vi "Main.vi"() -> ()   [LabVIEW 2023, in "QSM - Main.lvlib"]
uses:
  QSM - Main.lvlib
  Sched and Tubes.vi
  QSM - IODocs/IO Docs.vi
  LIMITS.vi
  QSM - Alarms/ALARMS.vi
  Controls/State Machine Message.ctl
  Controls/Message Queue Element Position.ctl
  UserCredentials.ctl
  Controls/biasdiff.ctl
  Controls/Event Handler Message.ctl
  <vilib>/event_ctls.llb/usereventprio.ctl
  QSM - Alarms/QSM - Alarms.lvlib
  QSM - IODocs/QSM - IODocs.lvlib
  Controls/gridvals.ctl
  QSM - Editor/QSM - Editor.lvlib
  QSM - Limits/QSM - Limits.lvlib
  Status.ctl
  Schedule.ctl
  Controls/stepvariables.ctl
  Controls/remoterdgs.ctl
  Controls/pulserdgs.ctl
  Controls/pulseparams.ctl
  Controls/cammeasures.ctl
  Controls/camdeflections.ctl
  Controls/camrefvals.ctl
  Controls/camexpvals.ctl
  Controls/camsettings.ctl
panel:
  out "Status 2":string="No Error"
  in  "PrintDatasheet":bool
  out "Status":T1
  out "Retest Select":bool[](array[boolean])
  out "Retest Step":u8
  in  "RetestEnd":bool
  in  "RetestOne":bool
  in  "FPCamera_PB":bool
  out "AIO Array Temp":dbl[](array[numeric])
  out "camsettings":T2
  out "current time":timestamp
  out "camrefs":T3
  out "deflections":T4
  out "cam measures":T5
  out "camexpvals":T6
  out "pulse params":T7
  out "pulse readings":T8
  out "Running":bool
  out "Sched Loaded":bool
  out "Tube Loaded":bool
  in  "Digital IO":bool[](array[boolean])
  out "Analog IO":dbl[](array[numeric])
  out "OffsetGain":dbl[](array[numeric])
  out "remrdgs":T9
  in  "Param Gx Only":cluster{"P06 G1 ONLY":bool, "P21 G2 ONLY":bool}
  in  "GXVALS":T10 {"g2rdggain" step=1e-05; "g2rdgoffset" step=1e-05; "g2spgain" step=1e-05; "g2spoffset" step=1e-05; "g1rdggain" step=1e-05; "g1rdgoffset" step=1e-05; "g1spgain" step=1e-05; "g1spoffset" step=1e-05}
  in  "BIAS DIFF":T11 {"DIFF" step=10.0; "BIAS" step=10.0}
  out "LIMITS":sgl[](array[numeric])
  in  "Run Results":i32(listbox)
  out "ALARM":bool
  out "PROC NOK":bool
  out "ALARMS":bool[](array[boolean])
  out "PROC OK":bool[](array[boolean])=[TRUE]
  out "STEP VARS":T12
  in  "PLC CURRENT STEP":u16 max=32
  in  "RESET Button":bool
  in  "RUN Button":bool
  in  "FINAL STEP":u16 max=32
  out "CURRENT STEP":u16 max=32
  in  "FIRST STEP":u16 max=32
  in  "ALARMS BUtton":bool
  in  "LIMITS Button":bool
  in  "IO/DOCS Button":bool
  in  "ENTER OP":string
  in  "ENTER SN":string
  in  "View Sched Button":bool
  in  "Schedule":T13 caption="Multicolumn Listbox"
  out "SchedNames[]":string[](array[string])
  out "SchedName":string
  out "SchedNum":string
  in  "sched sel Button":bool
  out "schd61-80":u32
  out "schd31-60":u32
  out "schd1-30":u32
  out "AP%":dbl
  out "T10":dbl
  out "T100":dbl
  out "HS":dbl
  out "RTC":dbl
  out "NAME":string
  out "TUBE":dbl
  in  "Load Tube Button":bool
  in  "Error In":errorcluster
  out "Error Out":errorcluster
  in  "Security Button":bool
  in  "stop":bool
  out "Access":u16
  out "Op Name":string
  out "BADGE NUMBER":string
  in  "Log In Button":bool
  in  "Editor Button":bool
  in  "User Creds":T14
  # "--STEP VARIABLES--"
  # "--CONTROLS--"
  # "--GRID TANK VALUES--"
  # "MCS-2093 Grid Tank\nFocal Spot Test Setup"
  # "XT229"
  # "ENTER SN"
  # "--CAMERA INTERFACE--"
  # "ENTER OP"
  # "REF"
  # "--READINGS--"
  # "Width"
  # "FrameRate"
  # "Mode"
  # "Length"
  # "--PULSE READINGS--"
  # "FW%max"
  # "X"
  # "Z"
  # "Y"
  # "MAG"
  # "pk"
  # "--STATUS--"
  # "**This Button Relaunches \nFLATPANELCAMERA application \nin event of crash/closure."
  # "OBpk"
  # "**Double Click Results Row \nto Select Retest Step**"
  # "FOCAL SPOT GRID TANK RUN RESULTS"
  # "OFFSET"
  # "OFFSET"
  # "GAIN"
  # "GAIN"
  # "OFFSET"
  # "OFFSET"
  # "GAIN"
  # "GAIN"
  # "STEP"
  # "NAME"
  # "NOTES"
  # "PARAMS"
  # "KV SP"
  # "MA/IF SP"
  # "EXP sec SP"
  # "COOL sec SP"
  # "scans.Mode"
  # "data item"
  # "min"
  # "max"
  # "init BIAS SP"
  # "init DIFF SP"
  # "max Gx"
  # "init EfDr SP"
  # "max Tries"
  # "TEST"
  # "LIM1"
  # "LIM2"
  # "LIM4"
  # "LIM3"
  # "CHAIN SCHEDS"
  # "RPTS"
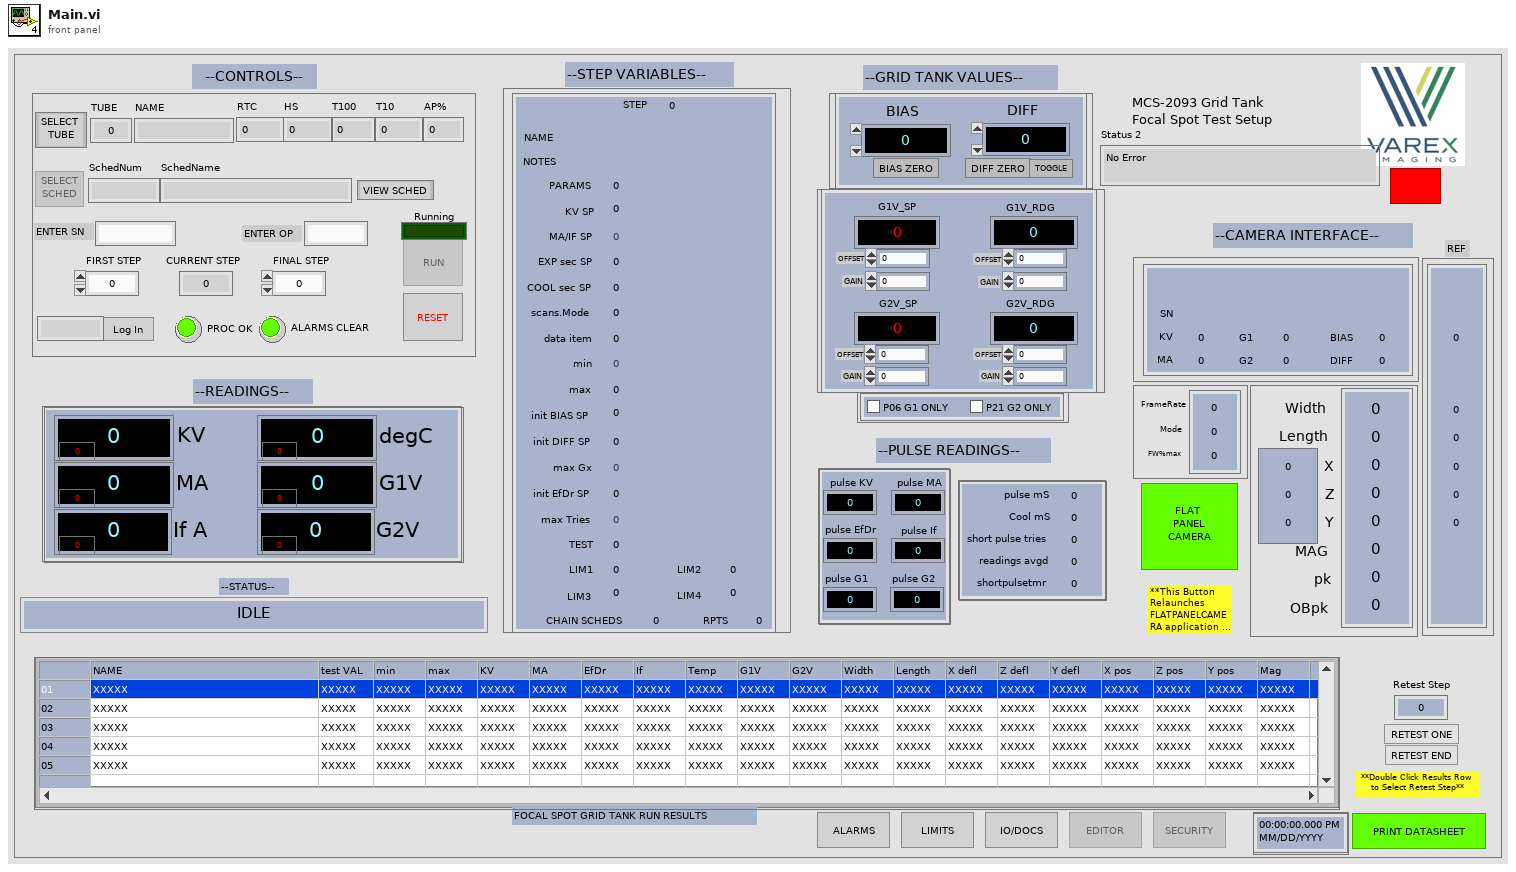
[diagram p1: front panel]
types:
  T1 = typedef "Status.ctl" = enum16{"IDLE", "RUN INITIATED", "RUNNING", "RESET INITIATED", "RESET", "RETESTING SELECTED STEP ONLY", "RETESTING SELECTED STEP TO END", "CAPTURING IMAGE", "WAITING FOR GRID SUPPLY", "WAITING FOR IMAGE", "ALARMS ACTIVE", "PROCNOK ACTIVE", "USER SIGNED ON", "TUBE SELECTED", "SCHEDULE SELECTED", "PRINTING DATASHEET", ""}
  T2 = typedef "QSM - Main.lvlib/camsettings.ctl" = cluster{"cam_FRAME_RATE":dbl, " cam_Mode":dbl, "cam_PERCENT_MAX":dbl}
  T3 = typedef "QSM - Main.lvlib/camrefvals.ctl" = cluster{"BIAS_ref":dbl, "cam_Wref":dbl, "cam_Lref":dbl, "cam_Xref":dbl, "cam_Zref":dbl, "cam_Yref":dbl}
  T4 = typedef "QSM - Main.lvlib/camdeflections.ctl" = cluster{"X_defl":dbl, "Y_defl":dbl, "Z_defl":dbl}
  T5 = typedef "QSM - Main.lvlib/cammeasures.ctl" = cluster{"cam_WIDTH":dbl, "cam_LENGTH":dbl, "cam_Xpos":dbl, "cam_Zpos":dbl, "cam_Ypos":dbl, "cam_MAG":dbl, "cam_PEAK":dbl, "cam_OB_pk":dbl}
  T6 = typedef "QSM - Main.lvlib/camexpvals.ctl" = cluster{"cam_IMAGE_PATH":string, "SN":string, "KV":dbl, "MA":dbl, "G1":dbl, "G2":dbl, "BIAS":dbl, "DIFF":dbl}
  T7 = typedef "QSM - Main.lvlib/pulseparams.ctl" = cluster{"pulse mS":dbl, "Cool mS":dbl, "short pulse tries":dbl, "readings avgd":dbl, "shortpulsetmr":dbl}
  T8 = typedef "QSM - Main.lvlib/pulserdgs.ctl" = cluster{"pulse EfDr":dbl, "pulse G1":dbl, "pulse G2":dbl, "pulse KV":dbl, "pulse MA":dbl, "pulse If":dbl}
  T9 = typedef "QSM - Main.lvlib/remoterdgs.ctl" = cluster{"remKVrdg":dbl, "remMArdg":dbl, "remIfArdg":dbl, "Temprdg":dbl, "G1Vrdg":dbl, "G2Vrdg":dbl, "remKVsp":dbl, "remMAsp":dbl, "remIfAsp":dbl, "Tempsp":dbl, "G1Vsp":dbl, "G2Vsp":dbl}
  T10 = typedef "QSM - Main.lvlib/gridvals.ctl" = cluster{"G1V_SP":dbl, "G2V_SP":dbl, "G1V_RDG":dbl, "G2V_RDG":dbl, "g1spoffset":dbl, "g1spgain":dbl, "g1rdgoffset":dbl, "g1rdggain":dbl, "g2spoffset":dbl, "g2spgain":dbl, "g2rdgoffset":dbl, "g2rdggain":dbl}
  T11 = typedef "QSM - Main.lvlib/biasdiff.ctl" = cluster{"BIAS":dbl, "BIAS_ZER":bool, "DIFF_ZER":bool, "DIFF_TOGGLE":bool, "DIFF":dbl}
  T12 = typedef "QSM - Main.lvlib/stepvariables.ctl" = cluster{"NAME":string, "NOTES":string, "PARAMS":u32, "KV  SP":dbl, "MA/IF  SP":dbl, "init BIAS SP":dbl, "max Gx":dbl, "TEST":u32, "min":dbl, "max":dbl, "LIM1":dbl, "LIM2":dbl, "LIM3":dbl, "LIM4":dbl, "data item":dbl, "chain scheds":dbl, "REPEATS":dbl, "STEP NUM":u32, "EXP s SP":dbl, "COOL s SP":dbl, "scans mode":dbl, "init EfDr":dbl, "max Tries":dbl, "init DIFF SP":dbl}
  T13 = typedef "Schedule.ctl" = i32
  T14 = typedef "UserCredentials.ctl" = cluster{"Badge Number":string, "Name":string, "Access":enum16{"", "Operator", "Admin", "Engineer"}}
  T15 = typedef "QSM - Main.lvlib/State Machine Message.ctl" = enum16{"Initialize", "Operator Signon", "Editor", "Security", "Select Tube", "Select Sched", "View Sched", "View IO/DOCS", "New Gx Val", "View LIMITS", "View ALARMS", "Start Step Change", "New Serial Number", "RUN Initiated", "RESET Initiated", "PLC Step Change", "RunResultRetestSelect", "Retest One", "Retest End", "PROC OK CHECK", "PROC NOK", "APIProcNOKUpdate", "APIAlarmsUpdate", "APILimitUpdate", "APIOperatorUpdate", "APIAnalogIOUpdate", "APIOffsetGainUpdate", "APIGXValsUpdate", "APIBiasDiffUpdate", "API Update Selected Tube", "API Update Selected Schedule", "ALARM CHECK", "ALARM ACTIVE", "CHECKS", "Print Datasheet", "FlatPanelCamera", "BIAS ZER", "DIFF ZER", "DIFF TOGGLE", "Handle Error", "Exit"}
  T16 = typedef "QSM - Main.lvlib/User Event Reference.ctl" = refnum<user-event>
  T17 = typedef "QSM - Main.lvlib/User Event Registration Reference.ctl" = refnum<event-registration>
  T18 = cluster{"Address IP":string, "Rack":i32, "Slot ":i32, "DB Number":i32, "Start":i32, "Amount":i32, "Word Length":i32}
  T19 = enum8{"Enabled", "Disabled", "Disabled and Grayed Out"}
  T20 = typedef "QSM - Main.lvlib/Message Queue Element Position.ctl" = enum16{"Front", "Back"}
  T21 = cluster{"Address IP":string, "Rack":i32, "Slot ":i32, "DB Number":i32, "Start":i32, "Amount":i32}
  T22 = typedef "usereventprio.ctl" = enum32{"high priority", "normal priority"}
  T23 = typedef "QSM - Main.lvlib/Event Handler Message.ctl" = enum16{"Exit"}
  T24 = cluster{"[0]":dbl, "[1]":dbl, "[2]":dbl, "[3]":dbl, "[4]":dbl, "[5]":dbl, "[6]":dbl, "[7]":dbl, "[8]":dbl, "[9]":dbl, "[10]":dbl, "[11]":dbl}
  T25 = cluster{"NAME":string, "NOTES":string, "PARAMS":u32, "KV  SP":dbl, "MA/IF  SP":dbl, "init BIAS SP":dbl, "max Gx":dbl, "TEST":u32, "min":dbl, "max":dbl, "LIM1":dbl, "LIM2":dbl, "LIM3":dbl, "LIM4":dbl, "data item":dbl, "chain scheds":dbl, "REPEATS":dbl, "STEP NUM":u32, "EXP s SP":dbl, "COOL s SP":dbl, "scans mode":dbl, "init EfDr":dbl, "max Tries":dbl, "init DIFF SP":dbl}
  T26 = cluster{"[0]":dbl, "[1]":dbl, "[2]":dbl, "[3]":dbl, "[4]":dbl, "[5]":dbl, "[6]":dbl, "[7]":dbl}
  T27 = enum32{"Bad", "Idle", "Run top level", "Running"}
  T28 = cluster{"Value[0]":dbl, "Value[1]":dbl, "Value[2]":dbl, "Value[3]":dbl, "Value[4]":dbl, "Value[5]":dbl, "Value[6]":dbl, "Value[7]":dbl, "Value[8]":dbl, "Value[9]":dbl, "Value[10]":dbl}
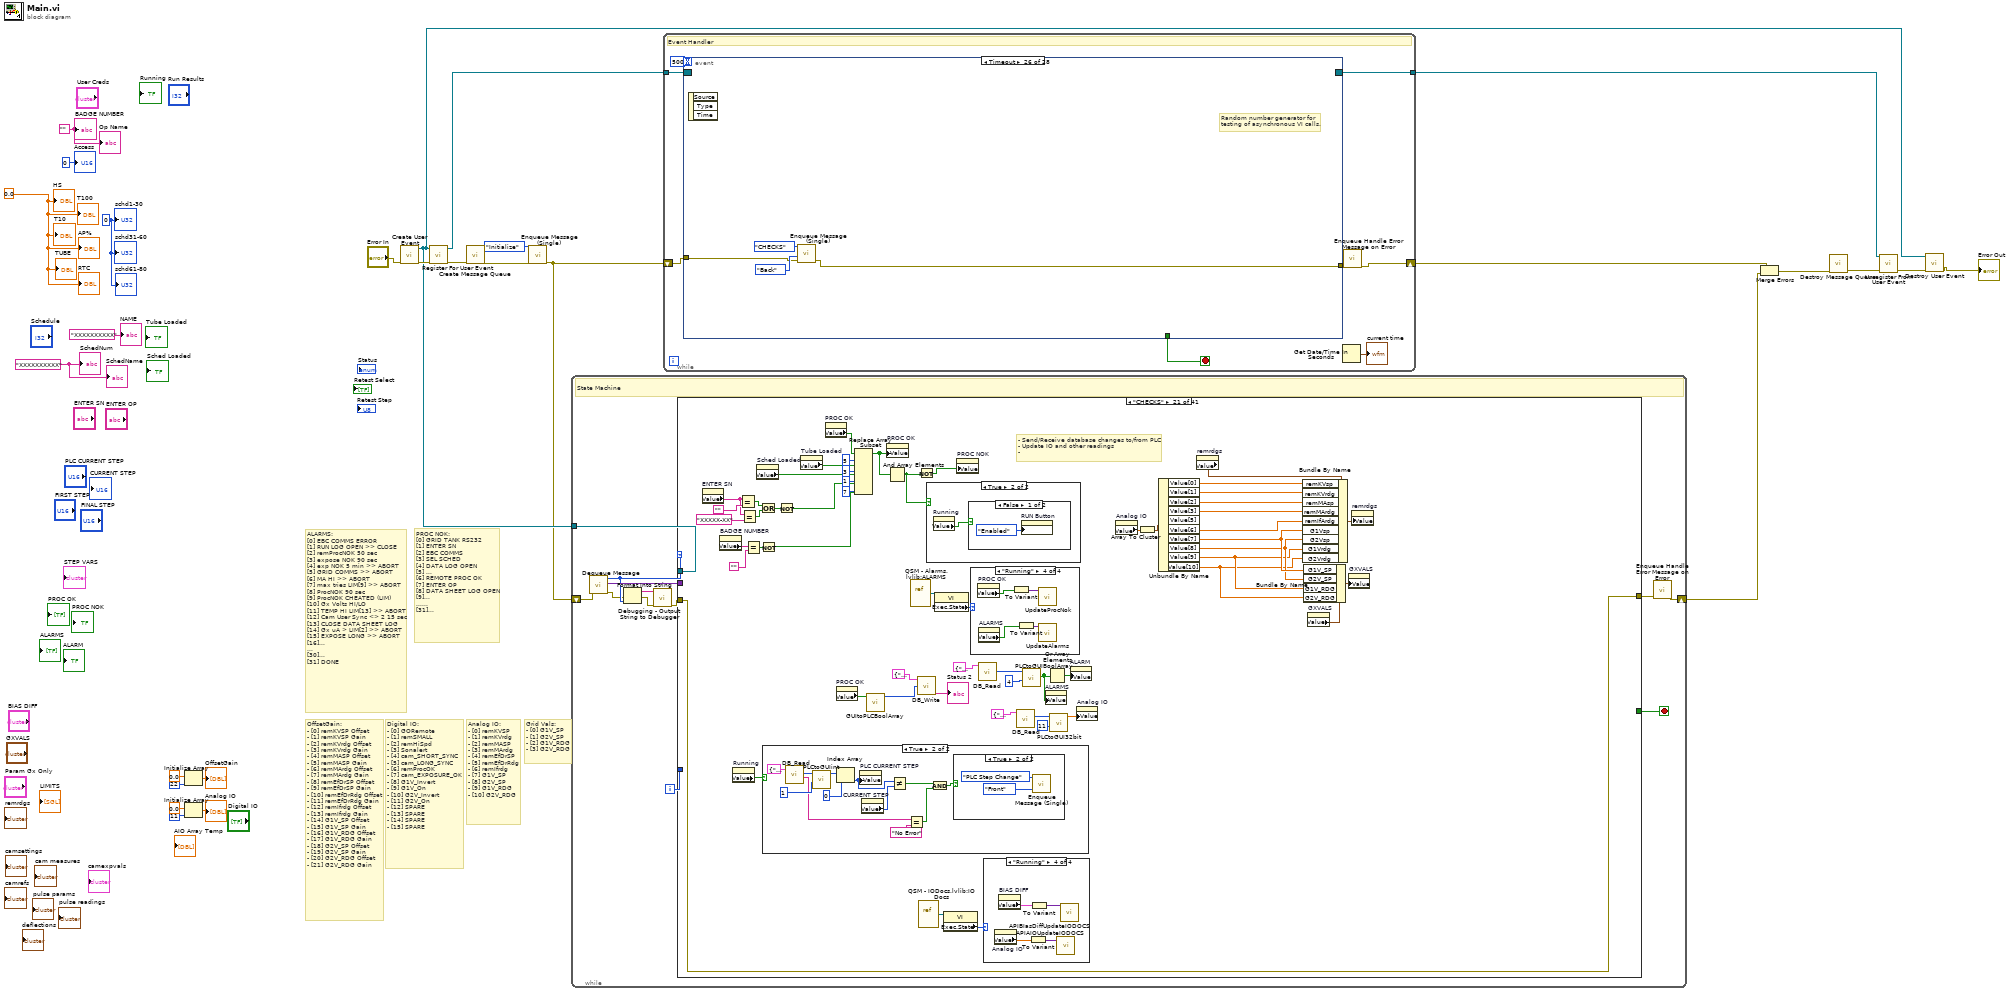
[diagram p0: block diagram]
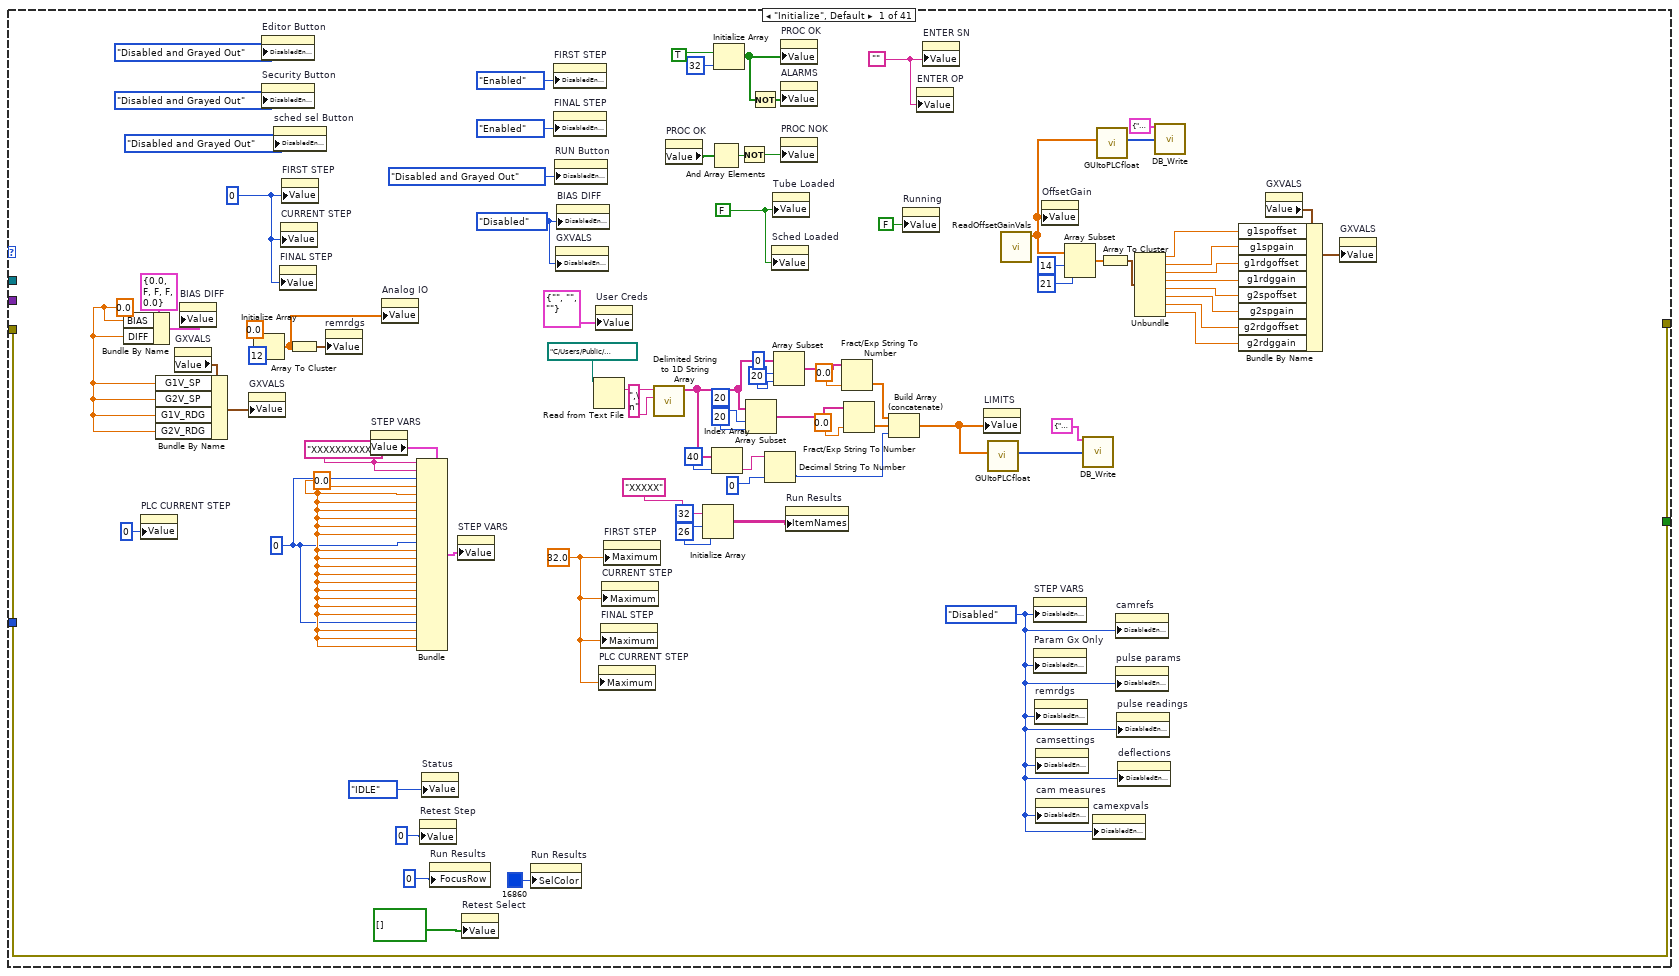
[diagram p2: hidden frame]
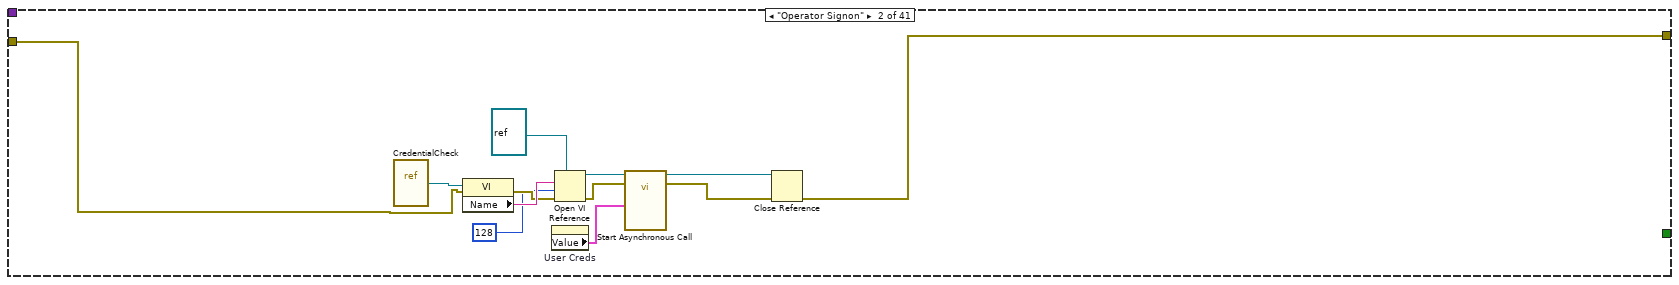
[diagram p3: hidden frame]
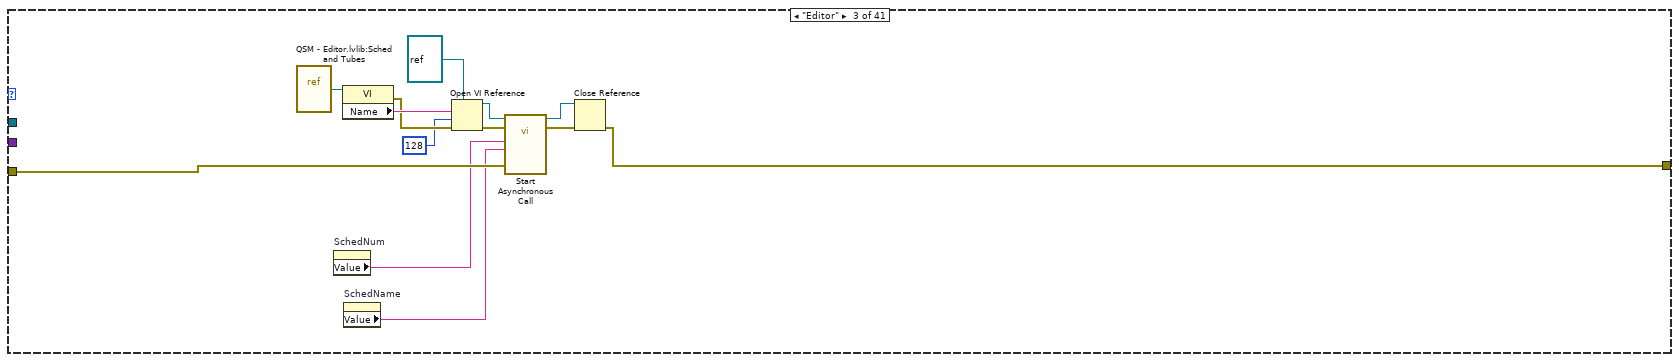
[diagram p4: hidden frame]
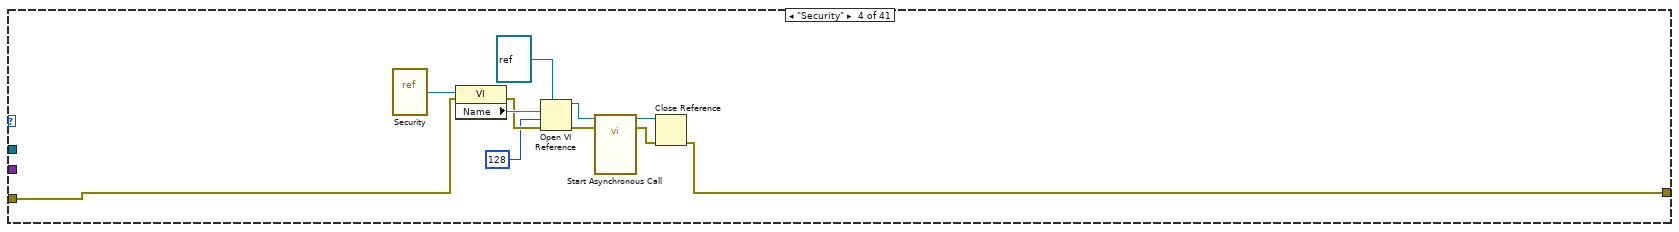
[diagram p5: hidden frame]
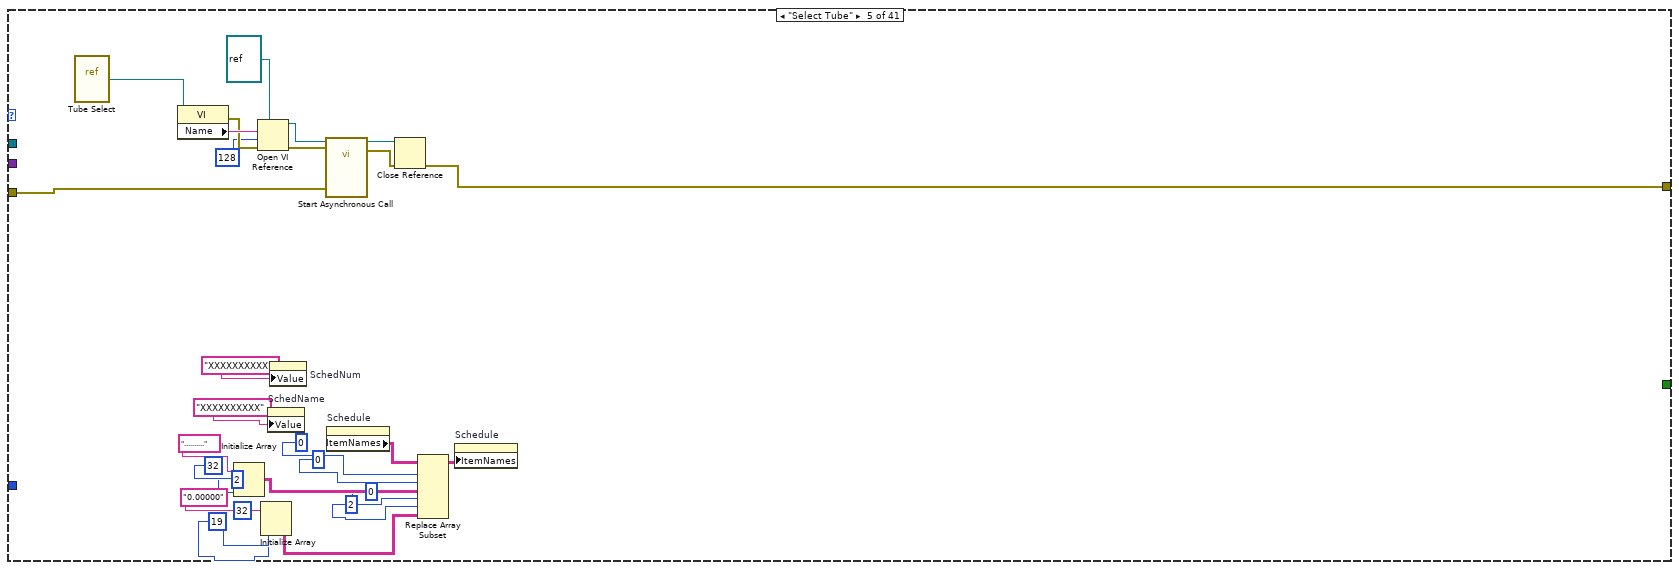
[diagram p6: hidden frame]
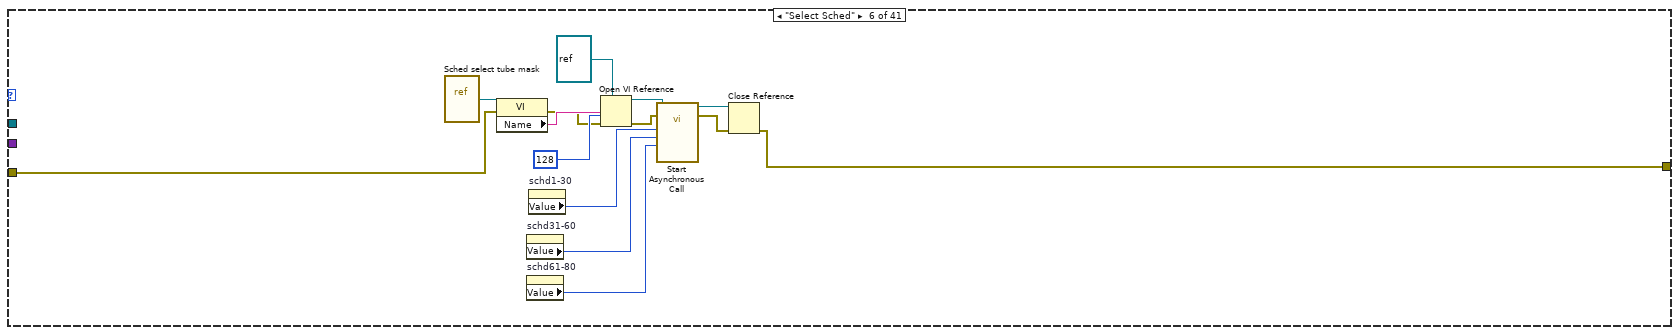
[diagram p7: hidden frame]
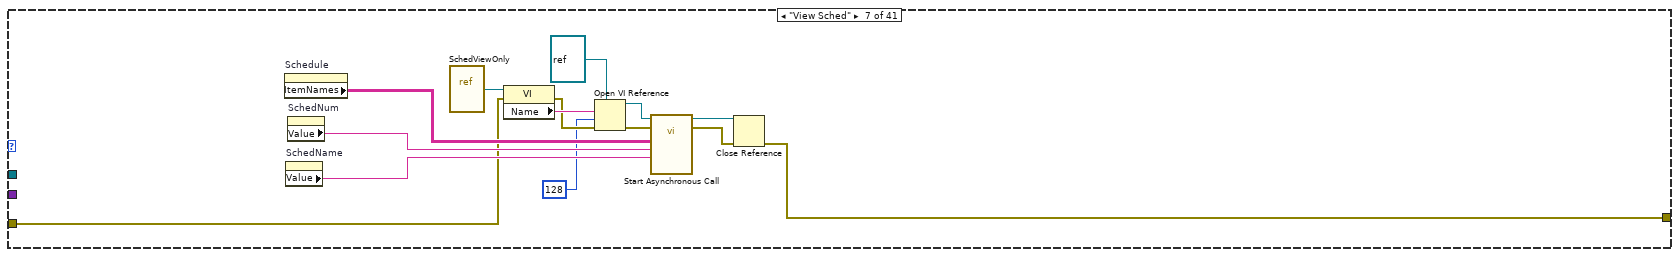
[diagram p8: hidden frame]
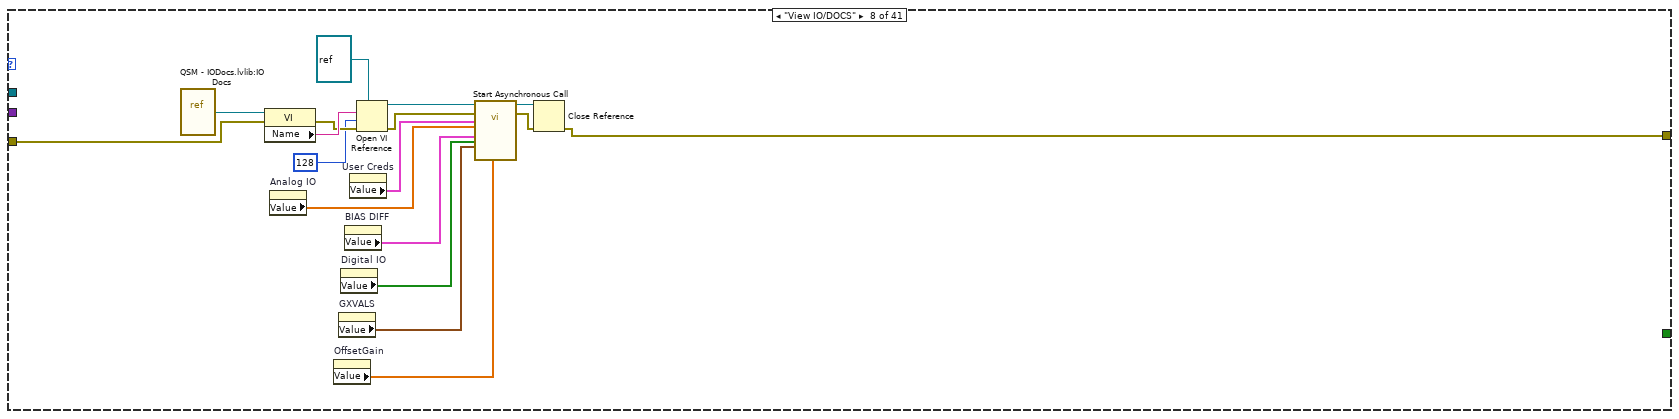
[diagram p9: hidden frame]
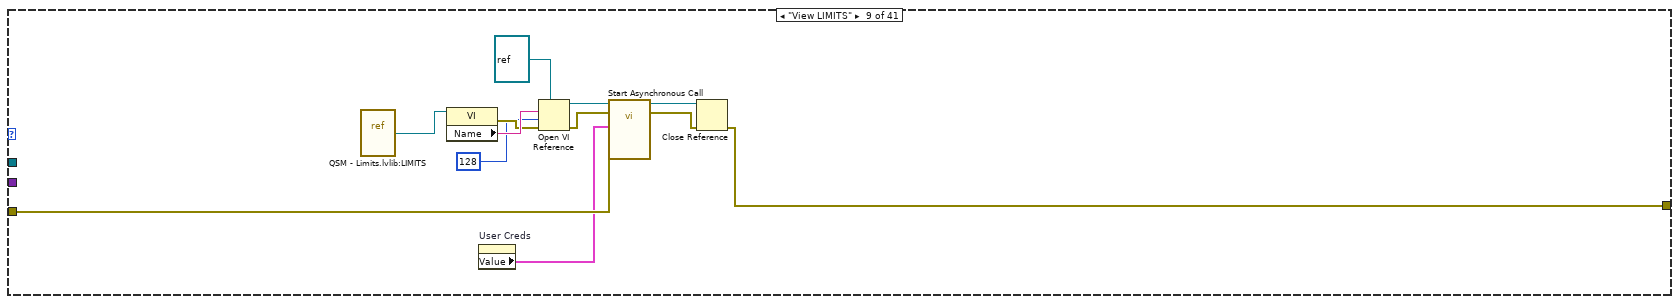
[diagram p10: hidden frame]
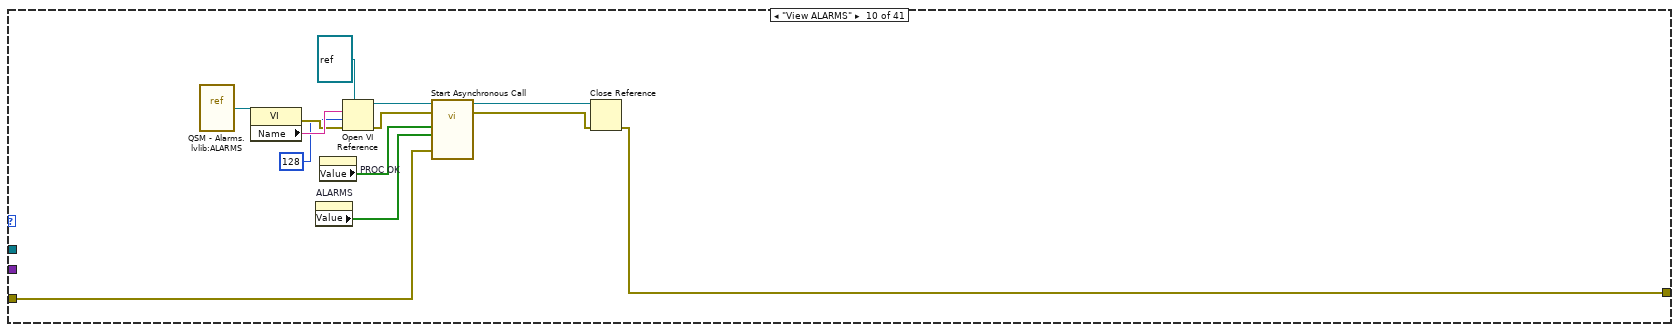
[diagram p11: hidden frame]
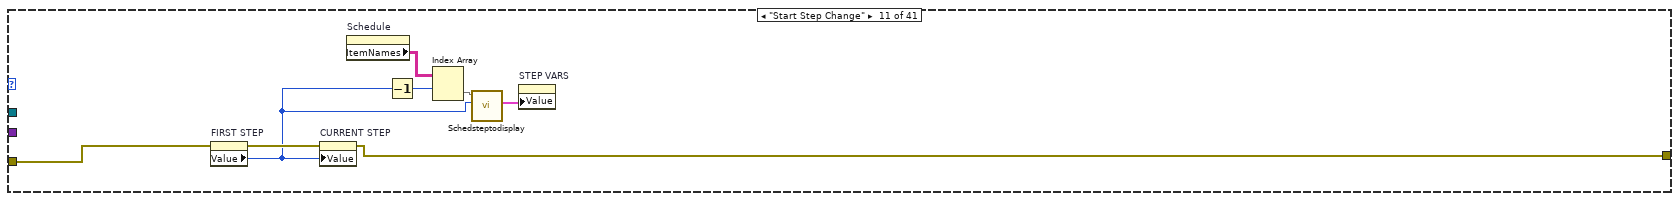
[diagram p12: hidden frame]
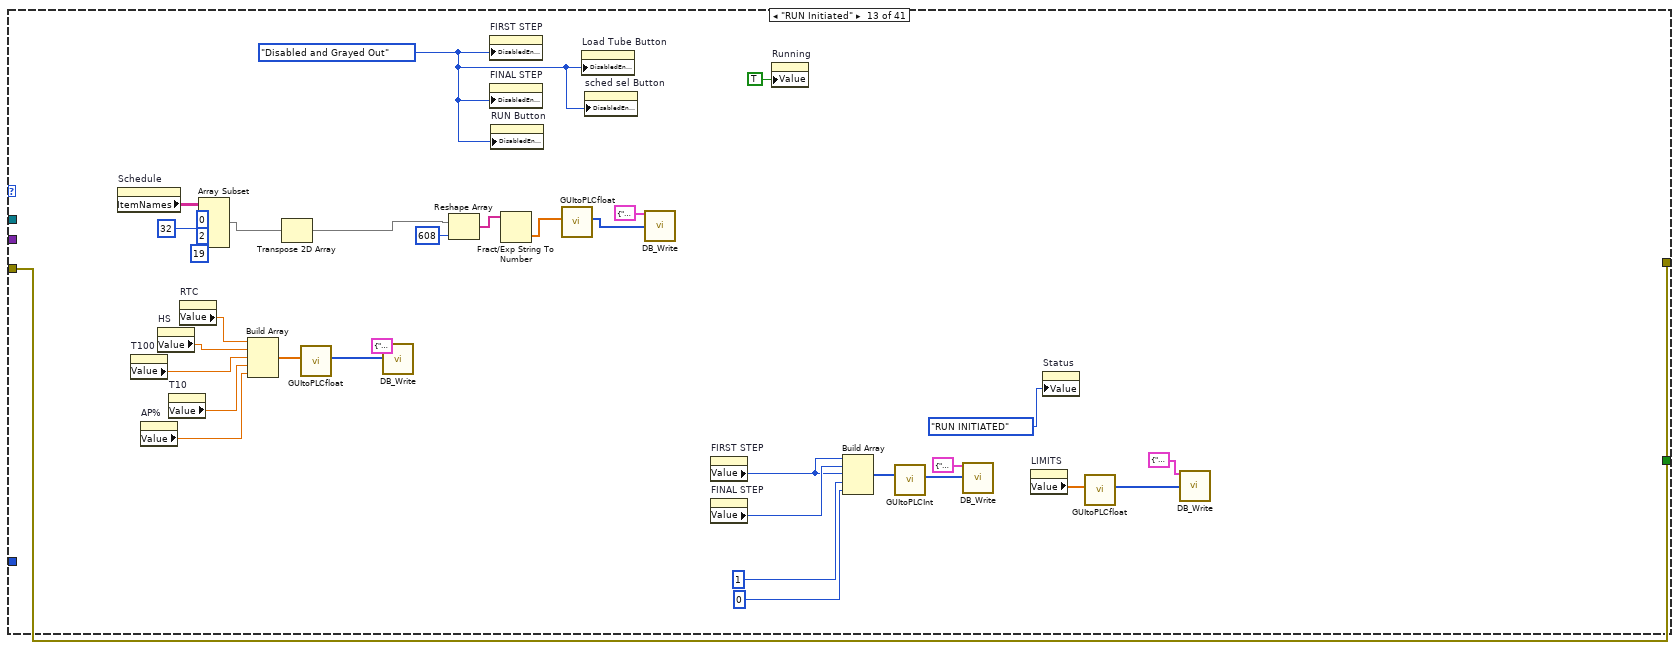
[diagram p14: hidden frame]
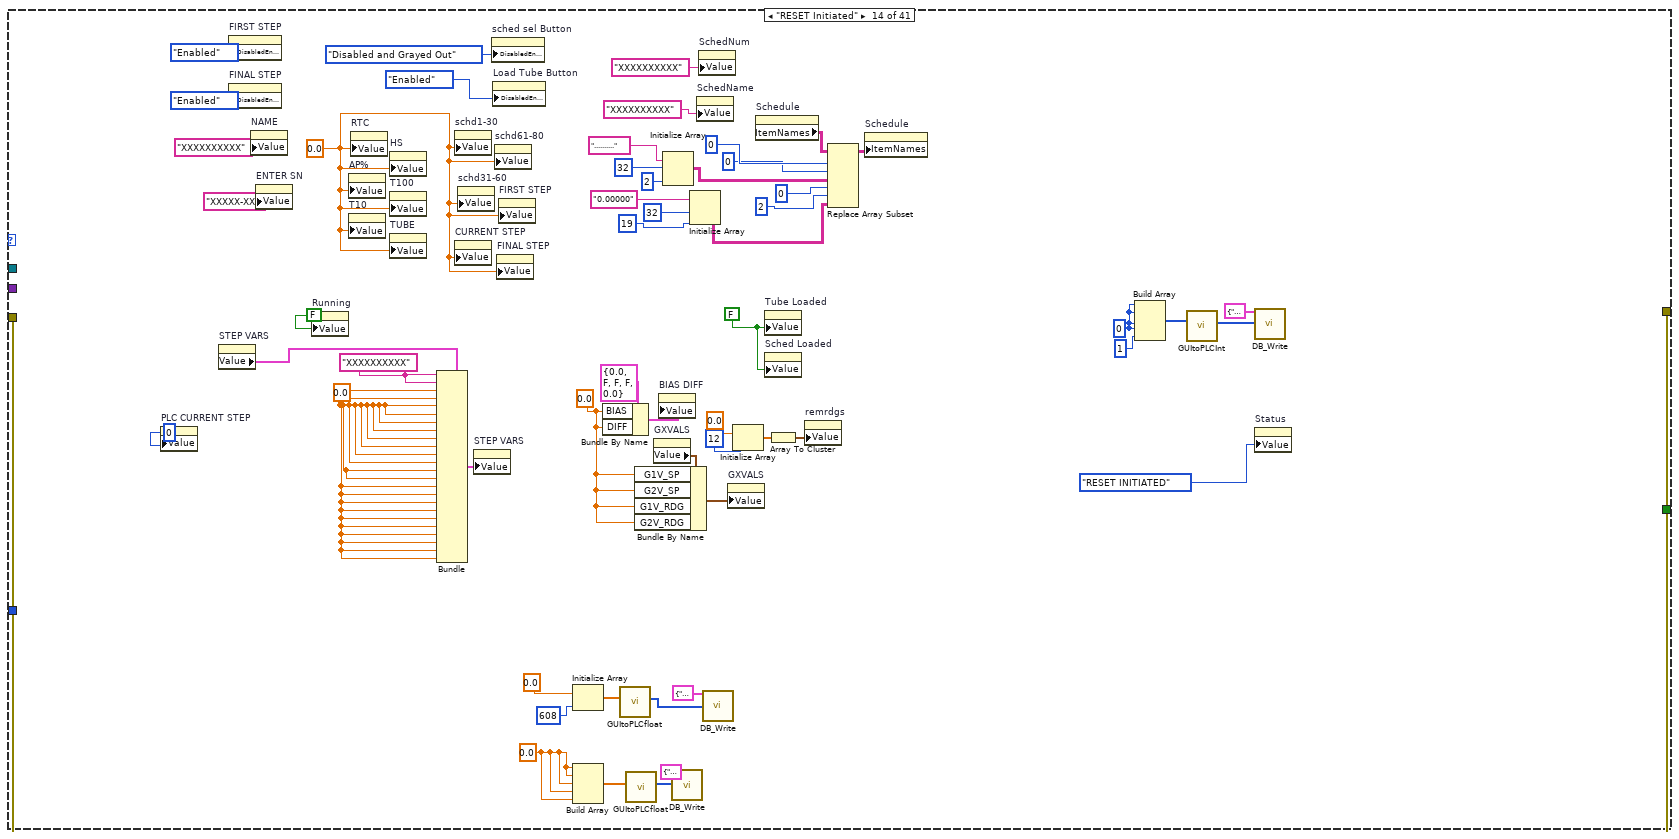
[diagram p15: hidden frame]
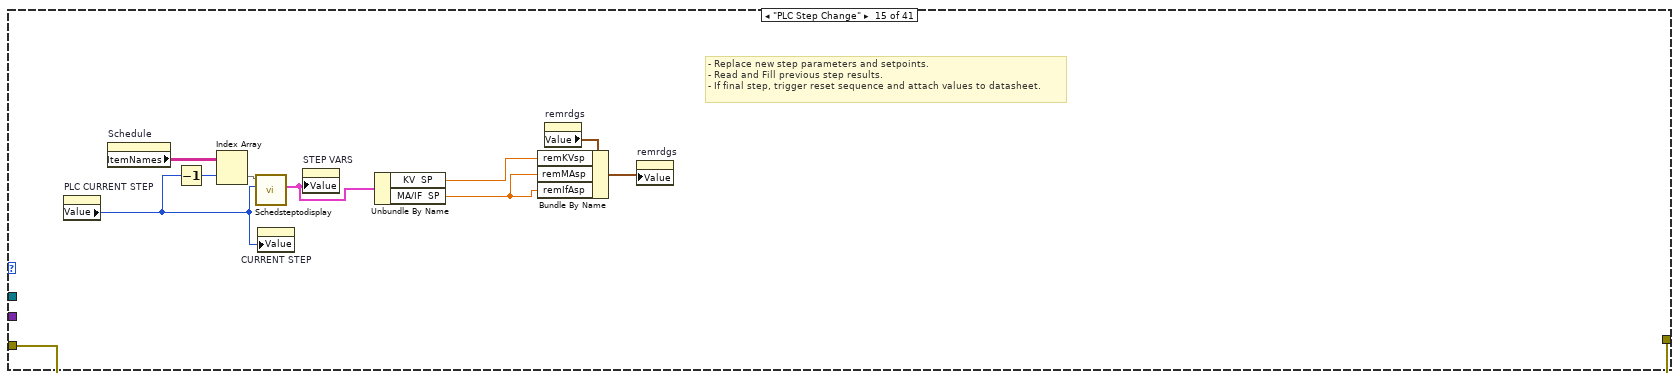
[diagram p16: hidden frame]
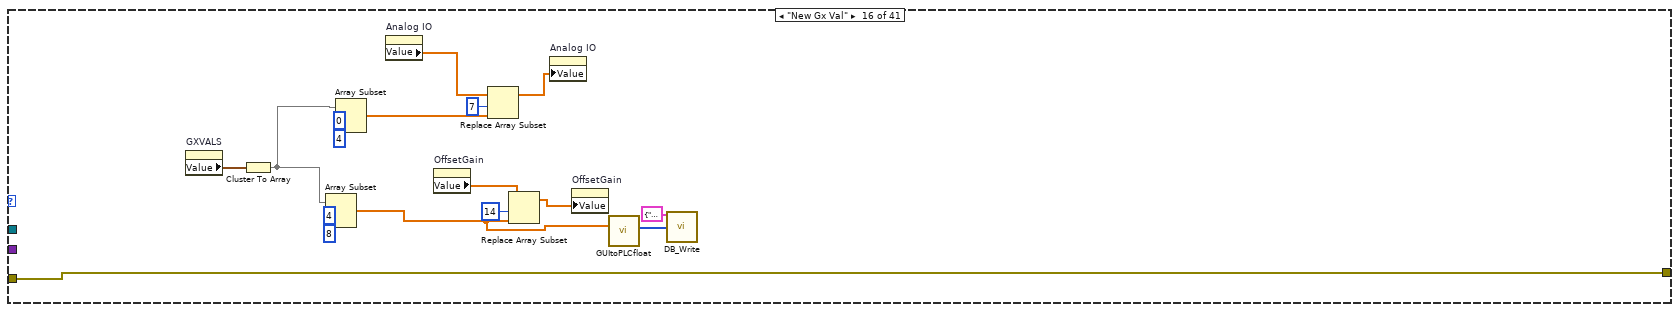
[diagram p17: hidden frame]
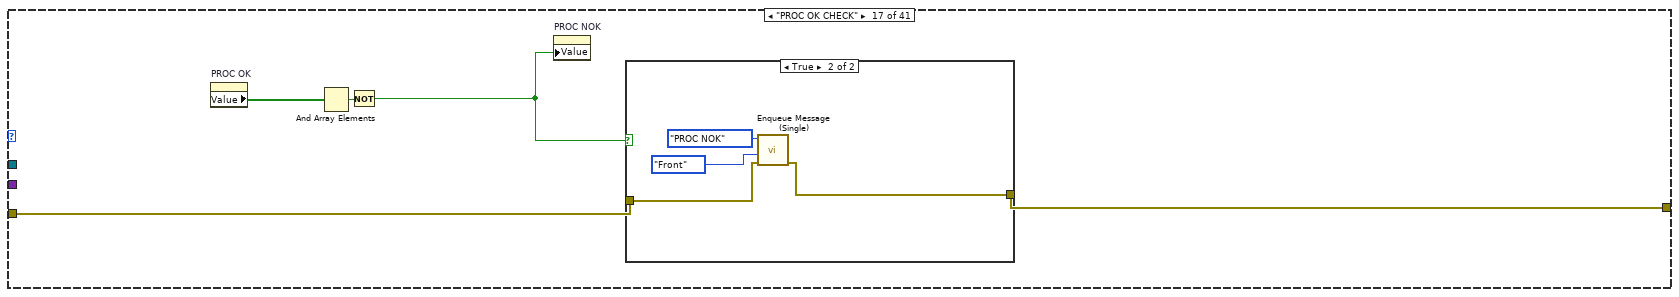
[diagram p18: hidden frame]
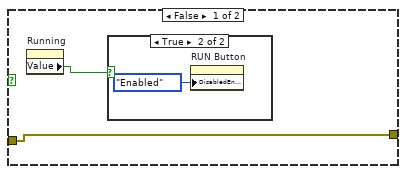
[diagram p19: hidden frame]
diagram:
  w18 = "XXXXXXXXXX" ("SchedNum")
  w19 = u32 0 ("schd1-30")
  w20 = 0.0 ("HS")
  w27 = "" ("Badge Number")
  # "Analog IO:\n- [0] remKVSP\n- [1] remKVrdg\n- [2] remMASP\n- [3] remMArdg\n- [4] remEfDrSP\n- [5] remEfDrRdg\n- [6] remIfrdg\n- [7] G1V_SP\n- [8] G2V_SP\n- [9] G1V_RDG\n- [10] G2V_RDG"
  # "OffsetGain:\n- [0] remKVSP Offset\n- [1] remKVSP Gain\n- [2] remKVrdg Offset\n- [3] remKVrdg Gain\n- [4] remMASP Offset\n- [5] remMASP Gain\n- [6] remMArdg Offset\n- [7] remMArdg Gain\n- [8] remEfDrSP Offset\n- [9] remEfDrSP Gain\n- [10] remEfDrRdg Offset\n- [11] remEfDrRdg Gain\n- [12] remIfrdg Offset\n- [13] remIfrdg Gain\n- [14] G1V_SP Offset\n- [15] G1V_SP Gain\n- [16] G1V_RDG Offset\n- [17] G1V_RDG Gain\n- [18] G2V_SP Offset\n- [19] G2V_SP Gain\n- [20] G2V_RDG Offset\n- [21] G2V_RDG Gain"
  # "Digital IO:\n- [0] GORemote\n- [1] remSMALL\n- [2] remHiSpd\n- [3] Sonalert\n- [4] cam_SHORT_SYNC\n- [5] cam_LONG_SYNC\n- [6] remProcOK\n- [7] cam_EXPOSURE_OK\n- [8] G1V_Invert\n- [9] G1V_On\n- [10] G2V_Invert\n- [11] G2V_On\n- [12] SPARE\n- [13] SPARE\n- [14] SPARE\n- [15] SPARE"
  # "Grid Vals:\n- [0] G1V_SP\n- [1] G2V_SP\n- [2] G1V_RDG\n- [3] G2V_RDG"
  # "PROC NOK:\n[0] GRID TANK RS232\n[1] ENTER SN\n[2] EBC COMMS\n[3] SEL SCHED\n[4] DATA LOG OPEN\n[5] ...\n[6] REMOTE PROC OK\n[7] ENTER OP\n[8] DATA SHEET LOG OPEN\n[9]...\n......\n[31]..."
  # "ALARMS:\n[0] EBC COMMS ERROR\n[1] RUN LOG OPEN >> CLOSE\n[2] remProcNOK 50 sec\n[3] expose NOK 90 sec\n[4] exp NOK 5 min >> ABORT\n[5] GRID COMMS >> ABORT\n[6] MA HI >> ABORT\n[7] max tries LIM[9] >> ABORT\n[8] ProcNOK 90 sec\n[9] ProcNOK CHEATED (LIM)\n[10] Gx Volts HI/LO\n[11] TEMP HI LIM[13] >> ABORT\n[12] Cam User Sync <> 2 15 sec\n[13] CLOSE DATA SHEET LOG\n[14] Gx uA > LIM[2] >> ABORT\n[15] EXPOSE LONG >> ABORT\n[16]...\n...\n[30]...\n[31] DONE"
  n1 = Initialize Array(0.0 ("element"), 22 ("dimension size")) -> (→"OffsetGain":dbl[])
  n2 = Initialize Array(0.0 ("element"), 11 ("dimension size")) -> (→"Analog IO":dbl[])
  n3 = call "Create User Event.vi"("Error In"="Error In") -> ("Error Out"=w17:errorcluster, "User Event Reference"=w9:T16)  [unwired: 9 in]
  n4 = call "Register For User Event.vi"("Error In"=w17, "User Event Reference"=w9) -> ("Error Out"=w15:errorcluster, "User Event Registration Reference"=w10:T17)  [unwired: 8 in]
  n5 = call "Create Message Queue.vi"("Error In"=w15) -> ("Error Out"=w1:errorcluster)  [unwired: 10 in]
  n6 = call "Enqueue Message (Single).vi"("Error In"=w1, "State Machine Message"=State_Machine_Message."Initialize") -> ("Error Out"=w8:errorcluster)  [unwired: 9 in]
  n7 = while {
    shift-right: [w37] -> w23
    shift-left: w8 -> [w35]
    tunnel: w9 -> [w34]
    i -> [w33]
    stop <- w36 stop-if-true
    # "State Machine"
    n8 = call "Dequeue Message.vi"("Error In"=w35) -> ("Error Out"=w31:errorcluster, "Data"=w39:variant, "State Machine Message"=w32:T15)  [unwired: 8 in]
    n9 = Format Into String(error in=w31, w32) -> (resulting string=w29:string, error out=w30:errorcluster)  [unwired: 2 in]
    n10 = call "Debugging - Output String to Debugger.vi"("Error In"=w30, "String"=w29) -> ("Error Out"=w28:errorcluster)  [unwired: 9 in]
    n11 = case shown="\"CHECKS\"" w32 {
      tunnel: w39 -> [_ _ _ _ _ _ _ _ _ _ _ _ _ _ _ _ _ _ _ _ _ w499 _ _ _ _ w519 w528 w545 w561 w587 _ w608 w613 w625 w681 w732 _ _ _ _]
      tunnel: w28 -> [w103 w125 w139 w150 w165 w188 w203 w216 w235 w247 w264 w265 w299 w351 w362 w368 w384 w397 w402 w412 w449 w497 w506 w509 w510 w514 w521 w529 w544 w560 w586 w588 w607 w612 w626 w680 w731 w741 w750 w754 w764]
      tunnel: [w103 w124 w138 w149 w160 w187 w202 w215 w234 w244 w262 w265 w299 w351 w362 w368 w383 w396 w401 w411 w449 w495 w504 w509 w510 w514 w520 w524 w543 w559 w580 w588 w605 w611 w615 w668 w730 w741 w750 w753 w764] -> w38
      tunnel: [_ _ _ _ _ _ _ _ _ _ _ _ _ _ _ _ _ _ _ _ _ _ TRUE _ _ _ _ _ _ _ _ _ _ _ _ _ _ _ _ _ _] -> w36
      tunnel: w34 -> [_ _ _ _ _ _ _ _ _ _ _ _ _ _ _ _ _ _ _ _ _ _ w503 _ _ _ _ _ _ _ _ _ _ _ _ _ _ _ _ _ _]
      tunnel: w33 -> [_ _ _ _ _ _ _ _ _ _ _ _ _ _ _ _ _ _ _ _ _ _ _ _ _ _ _ _ _ _ _ _ _ _ _ _ _ _ _ _ _]
      frame "Initialize", Default {
        w45 = T19."Disabled" ("Disabled")
        w68 = 32.0 ("Data Entry Limits:Maximum")
        w73 = 0.0 ("BIAS")
        w79 = ""
        w80 = FALSE ("Tube Loaded")
        w81 = T19."Disabled" ("Disabled")
        w84 = u32 0 ("PARAMS")
        w117 = 0.0
        w118 = "XXXXXXXXXX" ("NAME")
        w121 = 0 ("STARTING STEP")
        n12 = Bundle By Name(cluster=T11 {"BIAS"=0.0, "BIAS_ZER"=FALSE, "DIFF_ZER"=FALSE, "DIFF_TOGGLE"=FALSE, "DIFF"=0.0} ("BIAS DIFF"), "BIAS"=w73, "DIFF"=w73) -> (w77:T11)
        n13 = property on="PLC CURRENT STEP" class="DigNum (strict)"("Value"=u16 0 ("PLC CURRENT STEP 2")) -> ()  [unwired: 2 in, 2 out]
        n14 = property on="GXVALS" class="Clust (strict)"() -> ("Value"=w74:T10)  [unwired: 2 in, 2 out]
        n15 = Bundle By Name(cluster=w74, "G1V_SP"=w73, "G2V_SP"=w73, "G1V_RDG"=w73, "G2V_RDG"=w73) -> (w75:T10)
        n16 = property on="BIAS DIFF" class="Clust (strict)"("Value"=w77) -> ()  [unwired: 2 in, 2 out]
        n17 = property on="GXVALS" class="Clust (strict)"("Value"=w75) -> ()  [unwired: 2 in, 2 out]
        n18 = Initialize Array(0.0 ("element"), 12 ("dimension size")) -> (w69:dbl[])
        n19 = property on="Editor Button" class="Bool"("DisabledEnum"=T19."Disabled and Grayed Out" ("Disabled")) -> ()  [unwired: 2 in, 2 out]
        n20 = property on="Security Button" class="Bool (strict)"("DisabledEnum"=T19."Disabled and Grayed Out" ("Disabled")) -> ()  [unwired: 2 in, 2 out]
        n21 = property on="sched sel Button" class="Bool (strict)"("DisabledEnum"=T19."Disabled and Grayed Out" ("Disabled")) -> ()  [unwired: 2 in, 2 out]
        n22 = property on="FINAL STEP" class="DigNum (strict)"("Value"=w121) -> ()  [unwired: 2 in, 2 out]
        n23 = property on="CURRENT STEP" class="DigNum (strict)"("Value"=w121) -> ()  [unwired: 2 in, 2 out]
        n24 = property on="FIRST STEP" class="DigNum (strict)"("Value"=w121) -> ()  [unwired: 2 in, 2 out]
        n25 = Array To Cluster(array=w69) -> (cluster=w76:T24)
        n26 = property on="remrdgs" class="Clust (strict)"("Value"=w76) -> ()  [unwired: 2 in, 2 out]
        n27 = property on="STEP VARS" class="Clust (strict)"() -> ("Value"=w50:T25)  [unwired: 2 in, 2 out]
        n28 = property on="Analog IO" class="Arr (strict)"("Value"=w69) -> ()  [unwired: 2 in, 2 out]
        n29 = Bundle(cluster=w50, "NAME"=w118, "NOTES"=w118, "PARAMS"=w84, "KV  SP"=w117, "MA/IF  SP"=w117, "init BIAS SP"=w117, "max Gx"=w117, "TEST"=w117, "min"=w117, "max"=w117, "LIM1"=w84, "LIM2"=w117, "LIM3"=w117, "LIM4"=w117, "data item"=w117, "chain scheds"=w117, "REPEATS"=w117, "STEP NUM"=w117, "EXP s SP"=w117, "COOL s SP"=w117, "scans mode"=w84, "init EfDr"=w117, "max Tries"=w117, "init DIFF SP"=w117) -> (w49:T25)
        n30 = property on="Retest Step" class="DigNum (strict)"("Value"=u8 0 ("Retest Step")) -> ()  [unwired: 2 in, 2 out]
        n31 = property on="Status" class="Enum (strict)"("Value"=Status."IDLE" ("Status")) -> ()  [unwired: 2 in, 2 out]
        n32 = property on="Run Results" class="MCListbox (strict)"("FocusRow"=0 ("Focus Row")) -> ()  [unwired: 2 in, 2 out]
        n33 = property on="STEP VARS" class="Clust (strict)"("Value"=w49) -> ()  [unwired: 2 in, 2 out]
        n34 = property on="Retest Select" class="Arr (strict)"("Value"=bool[] [] ("Retest Select")) -> ()  [unwired: 2 in, 2 out]
        n35 = property on="Run Results" class="MCListbox (strict)"("SelColor"=u32 16860 ("Selection Color")) -> ()  [unwired: 2 in, 2 out]
        n36 = property on="FIRST STEP" class="DigNum (strict)"("DisabledEnum"=T19."Enabled" ("Disabled")) -> ()  [unwired: 2 in, 2 out]
        n37 = property on="FINAL STEP" class="DigNum (strict)"("DisabledEnum"=T19."Enabled" ("Disabled")) -> ()  [unwired: 2 in, 2 out]
        n38 = property on="RUN Button" class="Bool (strict)"("DisabledEnum"=T19."Disabled and Grayed Out" ("Disabled")) -> ()  [unwired: 2 in, 2 out]
        n39 = property on="GXVALS" class="Clust (strict)"("DisabledEnum"=w81) -> ()  [unwired: 2 in, 2 out]
        n40 = property on="BIAS DIFF" class="Clust (strict)"("DisabledEnum"=w81) -> ()  [unwired: 2 in, 2 out]
        n41 = Read from Text File(file (use dialog)=path "C:/Users/Public/Documents/Grid2093/LIMITS/LIMITS.txt") -> (text=w98:string)  [unwired: 3 in, 3 out]
        n42 = property on="User Creds" class="Clust (strict)"("Value"=T14 {"Badge Number"="", "Name"="", "Access"=enum.""} ("User Creds")) -> ()  [unwired: 2 in, 2 out]
        n43 = property on="PLC CURRENT STEP" class="DigNum (strict)"("Maximum"=w68) -> ()  [unwired: 2 in, 2 out]
        n44 = property on="FINAL STEP" class="DigNum (strict)"("Maximum"=w68) -> ()  [unwired: 2 in, 2 out]
        n45 = property on="CURRENT STEP" class="DigNum (strict)"("Maximum"=w68) -> ()  [unwired: 2 in, 2 out]
        n46 = property on="FIRST STEP" class="DigNum (strict)"("Maximum"=w68) -> ()  [unwired: 2 in, 2 out]
        n47 = call <vilib>:"Delimited String to 1D String Array.vi"("delimiter"=",\n", "delimited string"=w98) -> ("string array"=w101:string[])  [unwired: 9 in]
        n48 = property on="PROC OK" class="Arr (strict)"() -> ("Value"=w110:bool[])  [unwired: 2 in, 2 out]
        n49 = Initialize Array("XXXXX", 32 ("dimension size"), 26 ("dimension size")) -> (w104:string[][])
        n50 = And Array Elements(Boolean array=w110) -> (logical AND=w109:bool)
        n51 = Index Array(array=w101, index=40) -> (element=w102:string)
        n52 = Initialize Array(TRUE, 32 ("dimension size")) -> (w112:bool[])
        n53 = Not(x=w109) -> (.not. x?=w108:bool)
        n54 = Array Subset(array=w101, index=20, length=20) -> (w100:string[])
        n55 = Not(x=w112) -> (.not. x?=w111:bool[])
        n56 = Decimal String To Number(string=w102, default (0L)=u32 0 ("default (0 I32)")) -> (number=w85:u32)  [unwired: 1 in, 1 out]
        n57 = property on="Sched Loaded" class="Bool (strict)"("Value"=w80) -> ()  [unwired: 2 in, 2 out]
        n58 = property on="Tube Loaded" class="Bool (strict)"("Value"=w80) -> ()  [unwired: 2 in, 2 out]
        n59 = Array Subset(array=w101, index=0, length=20) -> (w99:string[])
        n60 = property on="PROC OK" class="Arr (strict)"("Value"=w112) -> ()  [unwired: 2 in, 2 out]
        n61 = property on="ALARMS" class="Arr (strict)"("Value"=w111) -> ()  [unwired: 2 in, 2 out]
        n62 = property on="PROC NOK" class="Bool (strict)"("Value"=w108) -> ()  [unwired: 2 in, 2 out]
        n63 = property on="Run Results" class="MCListbox (strict)"("ItemNames"=w104) -> ()  [unwired: 2 in, 2 out]
        n64 = Fract/Exp String To Number(string=w99, default (0 dbl)=sgl 0.0 ("default (0 DBL)")) -> (number=w87:sgl[])  [unwired: 2 in, 1 out]
        n65 = Fract/Exp String To Number(string=w100, default (0 dbl)=sgl 0.0 ("default (0 DBL)")) -> (number=w86:sgl[])  [unwired: 2 in, 1 out]
        n66 = Build Array (concatenate)(w87, w86, w85) -> (w51:sgl[])
        n67 = property on="Running" class="Bool (strict)"("Value"=FALSE ("Running")) -> ()  [unwired: 2 in, 2 out]
        n68 = property on="ENTER OP" class="Str"("Value"=w79) -> ()  [unwired: 2 in, 2 out]
        n69 = property on="ENTER SN" class="Str"("Value"=w79) -> ()  [unwired: 2 in, 2 out]
        n70 = property on="LIMITS" class="Arr (strict)"("Value"=w51) -> ()  [unwired: 2 in, 2 out]
        n71 = call "GUItoPLCfloat.vi"("Real Input Array"=w51) -> ("DB Output Array"=w53:u8[])  [unwired: 10 in]
        n72 = call "ReadOffsetGainVals.vi"() -> ("Array"=w46:dbl[])  [unwired: 10 in, 1 out]
        n73 = property on="STEP VARS" class="Clust (strict)"("DisabledEnum"=w45) -> ()  [unwired: 2 in, 2 out]
        n74 = property on="Param Gx Only" class="Clust (strict)"("DisabledEnum"=w45) -> ()  [unwired: 2 in, 2 out]
        n75 = property on="remrdgs" class="Clust (strict)"("DisabledEnum"=w45) -> ()  [unwired: 2 in, 2 out]
        n76 = property on="camsettings" class="Clust (strict)"("DisabledEnum"=w45) -> ()  [unwired: 2 in, 2 out]
        n77 = property on="cam measures" class="Clust (strict)"("DisabledEnum"=w45) -> ()  [unwired: 2 in, 2 out]
        n78 = property on="OffsetGain" class="Arr (strict)"("Value"=w46) -> ()  [unwired: 2 in, 2 out]
        n79 = Array Subset(array=w46, index=14, length=21) -> (w65:dbl[])
        n80 = call "DB_Write.vi"("Input Params"=T18 {"Address IP"="192.168.10.80", "Rack"=0, "Slot "=0, "DB Number"=6, "Start"=0, "Amount"=160, "Word Length"=2}, "Array"=w53) -> ()  [unwired: 13 in, 1 out]
        n81 = property on="camexpvals" class="Clust (strict)"("DisabledEnum"=w45) -> ()  [unwired: 2 in, 2 out]
        n82 = call "GUItoPLCfloat.vi"("Real Input Array"=w46) -> ("DB Output Array"=w48:u8[])  [unwired: 10 in]
        n83 = Array To Cluster(array=w65) -> (cluster=w62:T26)
        n84 = property on="camrefs" class="Clust (strict)"("DisabledEnum"=w45) -> ()  [unwired: 2 in, 2 out]
        n85 = property on="pulse params" class="Clust (strict)"("DisabledEnum"=w45) -> ()  [unwired: 2 in, 2 out]
        n86 = property on="pulse readings" class="Clust (strict)"("DisabledEnum"=w45) -> ()  [unwired: 2 in, 2 out]
        n87 = property on="deflections" class="Clust (strict)"("DisabledEnum"=w45) -> ()  [unwired: 2 in, 2 out]
        n88 = Unbundle(w62) -> ("[0]"=w61:dbl, "[1]"=w60:dbl, "[2]"=w59:dbl, "[3]"=w58:dbl, "[4]"=w57:dbl, "[5]"=w56:dbl, "[6]"=w55:dbl, "[7]"=w54:dbl)
        n89 = call "DB_Write.vi"("Input Params"=T18 {"Address IP"="192.168.10.80", "Rack"=0, "Slot "=0, "DB Number"=12, "Start"=0, "Amount"=88, "Word Length"=2}, "Array"=w48) -> ()  [unwired: 13 in, 1 out]
        n90 = property on="GXVALS" class="Clust (strict)"() -> ("Value"=w64:T10)  [unwired: 2 in, 2 out]
        n91 = Bundle By Name(cluster=w64, "g1spoffset"=w61, "g1spgain"=w60, "g1rdgoffset"=w59, "g1rdggain"=w58, "g2spoffset"=w57, "g2spgain"=w56, "g2rdgoffset"=w55, "g2rdggain"=w54) -> (w63:T10)
        n92 = property on="GXVALS" class="Clust (strict)"("Value"=w63) -> ()  [unwired: 2 in, 2 out]
      }
      frame "Operator Signon" {
        n93 = vi-ref "CredentialCheck.vi"() -> (w128:refnum<vi>)
        n94 = property class="VI"(reference=w128, error in=w125) -> (error out=w134:errorcluster, "Name"=w135:string)  [unwired: 1 out]
        n95 = property on="User Creds" class="Clust (strict)"() -> ("Value"=w126:T14)  [unwired: 2 in, 2 out]
        n96 = Open VI Reference(type specifier VI Refnum (for type only)=refnum<vi> refnum, vi path=w135, options=128, error in (no error)=w134) -> (vi reference=w133:refnum<vi>, error out=w132:errorcluster)  [unwired: 2 in]
        n97 = call-by-ref "Start Asynchronous Call"(reference=w133, error in=w132, "User Creds"=w126) -> (reference out=w130:refnum<vi>, error out=w129:errorcluster)  [unwired: 8 in, 3 out]
        n98 = Close Reference(reference=w130, error in (no error)=w129) -> (error out=w124:errorcluster)
      }
      frame "Editor" {
        n99 = vi-ref "QSM - Editor.lvlib:Sched and Tubes.vi"() -> (w148:refnum<vi>)
        n100 = property on="SchedNum" class="Str"() -> ("Value"=w137:string)  [unwired: 2 in, 2 out]
        n101 = property class="VI"(reference=w148) -> (error out=w146:errorcluster, "Name"=w147:string)  [unwired: 1 in, 1 out]
        n102 = property on="SchedName" class="Str"() -> ("Value"=w136:string)  [unwired: 2 in, 2 out]
        n103 = Open VI Reference(type specifier VI Refnum (for type only)=refnum<vi> refnum, vi path=w147, options=128, error in (no error)=w146) -> (vi reference=w142:refnum<vi>, error out=w143:errorcluster)  [unwired: 2 in]
        n104 = call-by-ref "Start Asynchronous Call"(reference=w142, error in=w143, "Error In"=w139, "Preselected sched name"=w136, "Preselected sched"=w137) -> (reference out=w140:refnum<vi>, error out=w141:errorcluster)  [unwired: 8 in, 1 out]
        n105 = Close Reference(reference=w140, error in (no error)=w141) -> (error out=w138:errorcluster)
      }
      frame "Security" {
        n106 = vi-ref "Security.vi"() -> (w159:refnum<vi>)
        n107 = property class="VI"(reference=w159, error in=w150) -> (error out=w157:errorcluster, "Name"=w158:string)  [unwired: 1 out]
        n108 = Open VI Reference(type specifier VI Refnum (for type only)=refnum<vi> refnum, vi path=w158, options=128, error in (no error)=w157) -> (vi reference=w154:refnum<vi>, error out=w155:errorcluster)  [unwired: 2 in]
        n109 = call-by-ref "Start Asynchronous Call"(reference=w154, error in=w155) -> (reference out=w152:refnum<vi>, error out=w151:errorcluster)  [unwired: 11 in, 1 out]
        n110 = Close Reference(reference=w152, error in (no error)=w151) -> (error out=w149:errorcluster)
      }
      frame "Select Tube" {
        n111 = vi-ref "Tube Select.vi"() -> (w170:refnum<vi>)
        n112 = property class="VI"(reference=w170) -> (error out=w168:errorcluster, "Name"=w169:string)  [unwired: 1 in, 1 out]
        n113 = Initialize Array("..........", 32 ("dimension size"), 2 ("dimension size")) -> (w182:string[][])
        n114 = Open VI Reference(type specifier VI Refnum (for type only)=refnum<vi> refnum, vi path=w169, options=128, error in (no error)=w168) -> (vi reference=w163:refnum<vi>, error out=w164:errorcluster)  [unwired: 2 in]
        n115 = Initialize Array("0.00000", 32 ("dimension size"), 19 ("dimension size")) -> (w181:string[][])
        n116 = property on="SchedName" class="Str"("Value"="XXXXXXXXXX" ("SchedNum")) -> ()  [unwired: 2 in, 2 out]
        n117 = property on="SchedNum" class="Str"("Value"="XXXXXXXXXX" ("SchedNum")) -> ()  [unwired: 2 in, 2 out]
        n118 = call-by-ref "Start Asynchronous Call"(reference=w163, error in=w164, 8:"error in (no error)"=w165) -> (reference out=w162:refnum<vi>, error out=w161:errorcluster)  [unwired: 7 in, 4 out]
        n119 = property on="Schedule" class="MCListbox (strict)"() -> ("ItemNames"=w184:string[][])  [unwired: 2 in, 2 out]
        n120 = Close Reference(reference=w162, error in (no error)=w161) -> (error out=w160:errorcluster)
        n121 = Replace Array Subset(array=w184, new element #1=w182, index (row) #1=0 ("index"), index (col) #1=0 ("disabled index (col)"), new element #2=w181, index (row) #2=0 ("index"), index (col) #2=2 ("disabled index (col)")) -> (w183:string[][])
        n122 = property on="Schedule" class="MCListbox (strict)"("ItemNames"=w183) -> ()  [unwired: 2 in, 2 out]
      }
      frame "Select Sched" {
        n123 = vi-ref "Sched select tube mask.vi"() -> (w200:refnum<vi>)
        n124 = property class="VI"(reference=w200, error in=w188) -> (error out=w197:errorcluster, "Name"=w199:string)  [unwired: 1 out]
        n125 = property on="schd31-60" class="DigNum (strict)"() -> ("Value"=w190:u32)  [unwired: 2 in, 2 out]
        n126 = property on="schd61-80" class="DigNum (strict)"() -> ("Value"=w189:u32)  [unwired: 2 in, 2 out]
        n127 = property on="schd1-30" class="DigNum (strict)"() -> ("Value"=w191:u32)  [unwired: 2 in, 2 out]
        n128 = Open VI Reference(type specifier VI Refnum (for type only)=refnum<vi> refnum, vi path=w199, options=128, error in (no error)=w197) -> (vi reference=w196:refnum<vi>, error out=w195:errorcluster)  [unwired: 2 in]
        n129 = call-by-ref "Start Asynchronous Call"(reference=w196, error in=w195, "sched61-80mask"=w189, "sched31-60mask"=w190, "sched1-30mask"=w191) -> (reference out=w193:refnum<vi>, error out=w192:errorcluster)  [unwired: 6 in, 3 out]
        n130 = Close Reference(reference=w193, error in (no error)=w192) -> (error out=w187:errorcluster)
      }
      frame "View Sched" {
        n131 = property on="Schedule" class="MCListbox (strict)"() -> ("ItemNames"=w208:string[][])  [unwired: 2 in, 2 out]
        n132 = property on="SchedName" class="Str"() -> ("Value"=w206:string)  [unwired: 2 in, 2 out]
        n133 = property on="SchedNum" class="Str"() -> ("Value"=w207:string)  [unwired: 2 in, 2 out]
        n134 = vi-ref "SchedViewOnly.vi"() -> (w214:refnum<vi>)
        n135 = property class="VI"(reference=w214, error in=w203) -> (error out=w212:errorcluster, "Name"=w213:string)  [unwired: 1 out]
        n136 = Open VI Reference(type specifier VI Refnum (for type only)=refnum<vi> refnum, vi path=w213, options=128, error in (no error)=w212) -> (vi reference=w210:refnum<vi>, error out=w209:errorcluster)  [unwired: 2 in]
        n137 = call-by-ref "Start Asynchronous Call"(reference=w210, error in=w209, "schedname"=w206, "schednum"=w207, "SchedArray"=w208) -> (reference out=w205:refnum<vi>, error out=w204:errorcluster)  [unwired: 9 in]
        n138 = Close Reference(reference=w205, error in (no error)=w204) -> (error out=w202:errorcluster)
      }
      frame "View IO/DOCS" {
        n139 = vi-ref "QSM - IODocs.lvlib:IO Docs.vi"() -> (w225:refnum<vi>)
        n140 = property class="VI"(reference=w225, error in=w216) -> (error out=w230:errorcluster, "Name"=w231:string)  [unwired: 1 out]
        n141 = property on="Analog IO" class="Arr (strict)"() -> ("Value"=w222:dbl[])  [unwired: 2 in, 2 out]
        n142 = property on="OffsetGain" class="Arr (strict)"() -> ("Value"=w217:dbl[])  [unwired: 2 in, 2 out]
        n143 = property on="GXVALS" class="Clust (strict)"() -> ("Value"=w218:T10)  [unwired: 2 in, 2 out]
        n144 = property on="Digital IO" class="Arr (strict)"() -> ("Value"=w219:bool[])  [unwired: 2 in, 2 out]
        n145 = property on="BIAS DIFF" class="Clust (strict)"() -> ("Value"=w220:T11)  [unwired: 2 in, 2 out]
        n146 = property on="User Creds" class="Clust (strict)"() -> ("Value"=w221:T14)  [unwired: 2 in, 2 out]
        n147 = Open VI Reference(type specifier VI Refnum (for type only)=refnum<vi> refnum, vi path=w231, options=128, error in (no error)=w230) -> (vi reference=w223:refnum<vi>, error out=w229:errorcluster)  [unwired: 2 in]
        n148 = call-by-ref "Start Asynchronous Call"(reference=w223, error in=w229, "Analog IO"=w222, "BIAS DIFF"=w220, "Digital IO"=w219, "GXVALS Input"=w218, "User Creds"=w221, "OffsetGain"=w217) -> (reference out=w228:refnum<vi>, error out=w227:errorcluster)  [unwired: 9 in, 5 out]
        n149 = Close Reference(reference=w228, error in (no error)=w227) -> (error out=w215:errorcluster)
      }
      frame "View LIMITS" {
        n150 = vi-ref "QSM - Limits.lvlib:LIMITS.vi"() -> (w233:refnum<vi>)
        n151 = property class="VI"(reference=w233) -> (error out=w242:errorcluster, "Name"=w243:string)  [unwired: 1 in, 1 out]
        n152 = property on="User Creds" class="Clust (strict)"() -> ("Value"=w232:T14)  [unwired: 2 in, 2 out]
        n153 = Open VI Reference(type specifier VI Refnum (for type only)=refnum<vi> refnum, vi path=w243, options=128, error in (no error)=w242) -> (vi reference=w241:refnum<vi>, error out=w240:errorcluster)  [unwired: 2 in]
        n154 = call-by-ref "Start Asynchronous Call"(reference=w241, error in=w240, "Error In"=w235, "User Creds"=w232) -> (reference out=w238:refnum<vi>, error out=w237:errorcluster)  [unwired: 7 in, 3 out]
        n155 = Close Reference(reference=w238, error in (no error)=w237) -> (error out=w234:errorcluster)
      }
      frame "View ALARMS" {
        n156 = vi-ref "QSM - Alarms.lvlib:ALARMS.vi"() -> (w256:refnum<vi>)
        n157 = property class="VI"(reference=w256) -> (error out=w254:errorcluster, "Name"=w255:string)  [unwired: 1 in, 1 out]
        n158 = property on="ALARMS" class="Arr (strict)"() -> ("Value"=w250:bool[])  [unwired: 2 in, 2 out]
        n159 = property on="PROC OK" class="Arr (strict)"() -> ("Value"=w251:bool[])  [unwired: 2 in, 2 out]
        n160 = Open VI Reference(type specifier VI Refnum (for type only)=refnum<vi> refnum, vi path=w255, options=128, error in (no error)=w254) -> (vi reference=w252:refnum<vi>, error out=w249:errorcluster)  [unwired: 2 in]
        n161 = call-by-ref "Start Asynchronous Call"(reference=w252, error in=w249, "Error In"=w247, "ALARM Input"=w250, "PROC OK Input"=w251) -> (reference out=w246:refnum<vi>, error out=w245:errorcluster)  [unwired: 6 in, 3 out]
        n162 = Close Reference(reference=w246, error in (no error)=w245) -> (error out=w244:errorcluster)
      }
      frame "Start Step Change" {
        n163 = property on="FIRST STEP" class="DigNum (strict)"(error in=w264) -> (error out=w263:errorcluster, "Value"=w257:u16)  [unwired: 1 in, 1 out]
        n164 = property on="CURRENT STEP" class="DigNum (strict)"(error in=w263, "Value"=w257) -> (error out=w262:errorcluster)  [unwired: 1 in, 1 out]
        n165 = property on="Schedule" class="MCListbox (strict)"() -> ("ItemNames"=w259:string[][])  [unwired: 2 in, 2 out]
        n166 = Decrement(x=w257) -> (x-1=w258:u16)
        n167 = Index Array(array=w259, index (row)=w258) -> (element=w261:string[])  [unwired: 1 in]
        n168 = call "Schedsteptodisplay.vi"("step num"=w257, "step array"=w261) -> ("STEP VARS"=w260:T12)  [unwired: 9 in]
        n169 = property on="STEP VARS" class="Clust (strict)"("Value"=w260) -> ()  [unwired: 2 in, 2 out]
      }
      frame "New Serial Number" {
      }
      frame "RUN Initiated" {
        w298 = T19."Disabled and Grayed Out" ("Disabled")
        n170 = property on="Schedule" class="MCListbox (strict)"() -> ("ItemNames"=w296:string[][])  [unwired: 2 in, 2 out]
        n171 = property on="T100" class="DigNum (strict)"() -> ("Value"=w282:dbl)  [unwired: 2 in, 2 out]
        n172 = property on="AP%" class="DigNum (strict)"() -> ("Value"=w280:dbl)  [unwired: 2 in, 2 out]
        n173 = property on="HS" class="DigNum (strict)"() -> ("Value"=w283:dbl)  [unwired: 2 in, 2 out]
        n174 = property on="T10" class="DigNum (strict)"() -> ("Value"=w281:dbl)  [unwired: 2 in, 2 out]
        n175 = property on="RTC" class="DigNum (strict)"() -> ("Value"=w284:dbl)  [unwired: 2 in, 2 out]
        n176 = Array Subset(array=w296, index (row)=0 ("index"), length (row)=32 ("length"), index (col)=2 ("index"), length (col)=19 ("length")) -> (w290:string[][])
        n177 = Build Array(w284, w283, w282, w281, w280) -> (w279:dbl[])
        n178 = Transpose 2D Array(2D array=w290) -> (transposed array=w289:string[][])
        n179 = call "GUItoPLCfloat.vi"("Real Input Array"=w279) -> ("DB Output Array"=w277:u8[])  [unwired: 10 in]
        n180 = call "DB_Write.vi"("Input Params"=T18 {"Address IP"="192.168.10.80", "Rack"=0, "Slot "=0, "DB Number"=13, "Start"=0, "Amount"=20, "Word Length"=2}, "Array"=w277) -> ()  [unwired: 13 in, 1 out]
        n181 = Reshape Array(w289, 608 ("dimension size")) -> (w287:string[])
        n182 = property on="FIRST STEP" class="DigNum (strict)"("DisabledEnum"=w298) -> ()  [unwired: 2 in, 2 out]
        n183 = property on="FINAL STEP" class="DigNum (strict)"("DisabledEnum"=w298) -> ()  [unwired: 2 in, 2 out]
        n184 = property on="RUN Button" class="Bool (strict)"("DisabledEnum"=w298) -> ()  [unwired: 2 in, 2 out]
        n185 = Fract/Exp String To Number(string=w287) -> (number=w286:dbl[])  [unwired: 3 in, 1 out]
        n186 = call "GUItoPLCfloat.vi"("Real Input Array"=w286) -> ("DB Output Array"=w285:u8[])  [unwired: 10 in]
        n187 = property on="Load Tube Button" class="Bool (strict)"("DisabledEnum"=w298) -> ()  [unwired: 2 in, 2 out]
        n188 = property on="sched sel Button" class="Bool (strict)"("DisabledEnum"=w298) -> ()  [unwired: 2 in, 2 out]
        n189 = call "DB_Write.vi"("Input Params"=T18 {"Address IP"="192.168.10.80", "Rack"=0, "Slot "=0, "DB Number"=10, "Start"=0, "Amount"=2432, "Word Length"=2}, "Array"=w285) -> ()  [unwired: 13 in, 1 out]
        n190 = property on="FIRST STEP" class="DigNum (strict)"() -> ("Value"=w267:u16)  [unwired: 2 in, 2 out]
        n191 = property on="FINAL STEP" class="DigNum (strict)"() -> ("Value"=w276:u16)  [unwired: 2 in, 2 out]
        n192 = property on="Running" class="Bool (strict)"("Value"=TRUE ("Running")) -> ()  [unwired: 2 in, 2 out]
        n193 = Build Array(w267, w276, w267, u16 1 ("element"), u16 0 ("element")) -> (w273:u16[])
        n194 = call "GUItoPLCInt.vi"("Real Input Array"=w273) -> ("DB Output Array"=w271:u8[])  [unwired: 10 in]
        n195 = call "DB_Write.vi"("Input Params"=T18 {"Address IP"="192.168.10.80", "Rack"=0, "Slot "=0, "DB Number"=14, "Start"=0, "Amount"=10, "Word Length"=2}, "Array"=w271) -> ()  [unwired: 13 in, 1 out]
        n196 = property on="LIMITS" class="Arr (strict)"() -> ("Value"=w270:sgl[])  [unwired: 2 in, 2 out]
        n197 = property on="Status" class="Enum (strict)"("Value"=Status."RUN INITIATED" ("Status")) -> ()  [unwired: 2 in, 2 out]
        n198 = call "GUItoPLCfloat.vi"("Real Input Array"=w270) -> ("DB Output Array"=w269:u8[])  [unwired: 10 in]
        n199 = call "DB_Write.vi"("Input Params"=T18 {"Address IP"="192.168.10.80", "Rack"=0, "Slot "=0, "DB Number"=6, "Start"=0, "Amount"=160, "Word Length"=2}, "Array"=w269) -> ()  [unwired: 13 in, 1 out]
      }
      frame "RESET Initiated" {
        w303 = 0.0 ("element")
        w312 = u16 0 ("element")
        w318 = 0.0 ("BIAS")
        w327 = FALSE ("Tube Loaded")
        w328 = 0.0
        w329 = "XXXXXXXXXX" ("NAME")
        w333 = 0.0 ("RTC")
        n200 = property on="PLC CURRENT STEP" class="DigNum (strict)"("Value"=u16 0 ("PLC CURRENT STEP 2")) -> ()  [unwired: 2 in, 2 out]
        n201 = property on="STEP VARS" class="Clust (strict)"() -> ("Value"=w311:T12)  [unwired: 2 in, 2 out]
        n202 = property on="FIRST STEP" class="DigNum (strict)"("DisabledEnum"=T19."Enabled" ("Disabled")) -> ()  [unwired: 2 in, 2 out]
        n203 = property on="FINAL STEP" class="DigNum (strict)"("DisabledEnum"=T19."Enabled" ("Disabled")) -> ()  [unwired: 2 in, 2 out]
        n204 = property on="NAME" class="Str"("Value"="XXXXXXXXXX" ("NAME")) -> ()  [unwired: 2 in, 2 out]
        n205 = property on="ENTER SN" class="Str"("Value"="XXXXX-XX" ("ENTER SN")) -> ()  [unwired: 2 in, 2 out]
        n206 = property on="Running" class="Bool (strict)"("Value"=FALSE ("Running")) -> ()  [unwired: 2 in, 2 out]
        n207 = property on="AP%" class="DigNum (strict)"("Value"=w333) -> ()  [unwired: 2 in, 2 out]
        n208 = property on="T10" class="DigNum (strict)"("Value"=w333) -> ()  [unwired: 2 in, 2 out]
        n209 = property on="RTC" class="DigNum (strict)"("Value"=w333) -> ()  [unwired: 2 in, 2 out]
        n210 = property on="HS" class="DigNum (strict)"("Value"=w333) -> ()  [unwired: 2 in, 2 out]
        n211 = property on="T100" class="DigNum (strict)"("Value"=w333) -> ()  [unwired: 2 in, 2 out]
        n212 = property on="TUBE" class="DigNum (strict)"("Value"=w333) -> ()  [unwired: 2 in, 2 out]
        n213 = Bundle(cluster=w311, "NAME"=w329, "NOTES"=w329, "PARAMS"=w328, "KV  SP"=w328, "MA/IF  SP"=w328, "init BIAS SP"=w328, "max Gx"=w328, "TEST"=w328, "min"=w328, "max"=w328, "LIM1"=w328, "LIM2"=w328, "LIM3"=w328, "LIM4"=w328, "data item"=w328, "chain scheds"=w328, "REPEATS"=w328, "STEP NUM"=w328, "EXP s SP"=w328, "COOL s SP"=w328, "scans mode"=w328, "init EfDr"=w328, "max Tries"=w328, "init DIFF SP"=w328) -> (w310:T12)
        n214 = property on="schd1-30" class="DigNum (strict)"("Value"=w333) -> ()  [unwired: 2 in, 2 out]
        n215 = property on="CURRENT STEP" class="DigNum (strict)"("Value"=w333) -> ()  [unwired: 2 in, 2 out]
        n216 = property on="schd31-60" class="DigNum (strict)"("Value"=w333) -> ()  [unwired: 2 in, 2 out]
        n217 = property on="STEP VARS" class="Clust (strict)"("Value"=w310) -> ()  [unwired: 2 in, 2 out]
        n218 = property on="sched sel Button" class="Bool (strict)"("DisabledEnum"=T19."Disabled and Grayed Out" ("Disabled")) -> ()  [unwired: 2 in, 2 out]
        n219 = property on="Load Tube Button" class="Bool (strict)"("DisabledEnum"=T19."Enabled" ("Disabled")) -> ()  [unwired: 2 in, 2 out]
        n220 = property on="schd61-80" class="DigNum (strict)"("Value"=w333) -> ()  [unwired: 2 in, 2 out]
        n221 = property on="FINAL STEP" class="DigNum (strict)"("Value"=w333) -> ()  [unwired: 2 in, 2 out]
        n222 = property on="FIRST STEP" class="DigNum (strict)"("Value"=w333) -> ()  [unwired: 2 in, 2 out]
        n223 = Initialize Array(0.0 ("element"), 608 ("dimension size")) -> (w300:dbl[])
        n224 = Build Array(w303, w303, w303, w303, w303) -> (w307:dbl[])
        n225 = Bundle By Name(cluster=T11 {"BIAS"=0.0, "BIAS_ZER"=FALSE, "DIFF_ZER"=FALSE, "DIFF_TOGGLE"=FALSE, "DIFF"=0.0} ("BIAS DIFF"), "BIAS"=w318, "DIFF"=w318) -> (w326:T11)
        n226 = call "GUItoPLCfloat.vi"("Real Input Array"=w300) -> ("DB Output Array"=w308:u8[])  [unwired: 10 in]
        n227 = call "GUItoPLCfloat.vi"("Real Input Array"=w307) -> ("DB Output Array"=w306:u8[])  [unwired: 10 in]
        n228 = property on="GXVALS" class="Clust (strict)"() -> ("Value"=w317:T10)  [unwired: 2 in, 2 out]
        n229 = Bundle By Name(cluster=w317, "G1V_SP"=w318, "G2V_SP"=w318, "G1V_RDG"=w318, "G2V_RDG"=w318) -> (w319:T10)
        n230 = property on="BIAS DIFF" class="Clust (strict)"("Value"=w326) -> ()  [unwired: 2 in, 2 out]
        n231 = Initialize Array("..........", 32 ("dimension size"), 2 ("dimension size")) -> (w348:string[][])
        n232 = call "DB_Write.vi"("Input Params"=T18 {"Address IP"="192.168.10.80", "Rack"=0, "Slot "=0, "DB Number"=13, "Start"=0, "Amount"=20, "Word Length"=2}, "Array"=w306) -> ()  [unwired: 13 in, 1 out]
        n233 = Initialize Array("0.00000", 32 ("dimension size"), 19 ("dimension size")) -> (w347:string[][])
        n234 = property on="SchedName" class="Str"("Value"="XXXXXXXXXX" ("SchedNum")) -> ()  [unwired: 2 in, 2 out]
        n235 = property on="SchedNum" class="Str"("Value"="XXXXXXXXXX" ("SchedNum")) -> ()  [unwired: 2 in, 2 out]
        n236 = call "DB_Write.vi"("Input Params"=T18 {"Address IP"="192.168.10.80", "Rack"=0, "Slot "=0, "DB Number"=10, "Start"=0, "Amount"=2432, "Word Length"=2}, "Array"=w308) -> ()  [unwired: 13 in, 1 out]
        n237 = property on="GXVALS" class="Clust (strict)"("Value"=w319) -> ()  [unwired: 2 in, 2 out]
        n238 = Initialize Array(0.0 ("element"), 12 ("dimension size")) -> (w322:dbl[])
        n239 = property on="Schedule" class="MCListbox (strict)"() -> ("ItemNames"=w350:string[][])  [unwired: 2 in, 2 out]
        n240 = property on="Tube Loaded" class="Bool (strict)"("Value"=w327) -> ()  [unwired: 2 in, 2 out]
        n241 = property on="Sched Loaded" class="Bool (strict)"("Value"=w327) -> ()  [unwired: 2 in, 2 out]
        n242 = Array To Cluster(array=w322) -> (cluster=w321:T24)
        n243 = property on="remrdgs" class="Clust (strict)"("Value"=w321) -> ()  [unwired: 2 in, 2 out]
        n244 = Replace Array Subset(array=w350, new element #1=w348, index (row) #1=0 ("index"), index (col) #1=0 ("disabled index (col)"), new element #2=w347, index (row) #2=0 ("index"), index (col) #2=2 ("disabled index (col)")) -> (w349:string[][])
        n245 = property on="Schedule" class="MCListbox (strict)"("ItemNames"=w349) -> ()  [unwired: 2 in, 2 out]
        n246 = Build Array(w312, w312, w312, w312, u16 1 ("element")) -> (w315:u16[])
        n247 = call "GUItoPLCInt.vi"("Real Input Array"=w315) -> ("DB Output Array"=w313:u8[])  [unwired: 10 in]
        n248 = call "DB_Write.vi"("Input Params"=T18 {"Address IP"="192.168.10.80", "Rack"=0, "Slot "=0, "DB Number"=14, "Start"=0, "Amount"=10, "Word Length"=2}, "Array"=w313) -> ()  [unwired: 13 in, 1 out]
        n249 = property on="Status" class="Enum (strict)"("Value"=Status."RESET INITIATED" ("Status")) -> ()  [unwired: 2 in, 2 out]
      }
      frame "PLC Step Change" {
        # "- Replace new step parameters and setpoints.\n- Read and Fill previous step results.\n- If final step, trigger reset sequence and attach values to datasheet."
        n250 = property on="PLC CURRENT STEP" class="DigNum (strict)"() -> ("Value"=w355:u16)  [unwired: 2 in, 2 out]
        n251 = property on="Schedule" class="MCListbox (strict)"() -> ("ItemNames"=w364:string[][])  [unwired: 2 in, 2 out]
        n252 = Decrement(x=w355) -> (x-1=w361:u16)
        n253 = Index Array(array=w364, index (row)=w361) -> (element=w363:string[])  [unwired: 1 in]
        n254 = call "Schedsteptodisplay.vi"("step num"=w355, "step array"=w363) -> ("STEP VARS"=w356:T12)  [unwired: 9 in]
        n255 = property on="CURRENT STEP" class="DigNum (strict)"("Value"=w355) -> ()  [unwired: 2 in, 2 out]
        n256 = property on="STEP VARS" class="Clust (strict)"("Value"=w356) -> ()  [unwired: 2 in, 2 out]
        n257 = Unbundle By Name(w356) -> ("KV  SP"=w359:dbl, "MA/IF  SP"=w358:dbl)
        n258 = property on="remrdgs" class="Clust (strict)"() -> ("Value"=w360:T9)  [unwired: 2 in, 2 out]
        n259 = Bundle By Name(cluster=w360, "remKVsp"=w359, "remMAsp"=w358, "remIfAsp"=w358) -> (w357:T9)
        n260 = property on="remrdgs" class="Clust (strict)"("Value"=w357) -> ()  [unwired: 2 in, 2 out]
      }
      frame "New Gx Val" {
        n261 = property on="GXVALS" class="Clust (strict)"() -> ("Value"=w381:T10)  [unwired: 2 in, 2 out]
        n262 = Cluster To Array(cluster=w381) -> (array=w380:dbl[])
        n263 = Array Subset(array=w380, index=4, length=8) -> (w365:dbl[])
        n264 = Array Subset(array=w380, index=0, length=4) -> (w373:dbl[])
        n265 = property on="Analog IO" class="Arr (strict)"() -> ("Value"=w374:dbl[])  [unwired: 2 in, 2 out]
        n266 = property on="OffsetGain" class="Arr (strict)"() -> ("Value"=w375:dbl[])  [unwired: 2 in, 2 out]
        n267 = Replace Array Subset(array=w374, new element=w373, index=7) -> (w372:dbl[])
        n268 = Replace Array Subset(array=w375, new element=w365, index=14) -> (w369:dbl[])
        n269 = property on="Analog IO" class="Arr (strict)"("Value"=w372) -> ()  [unwired: 2 in, 2 out]
        n270 = property on="OffsetGain" class="Arr (strict)"("Value"=w369) -> ()  [unwired: 2 in, 2 out]
        n271 = call "GUItoPLCfloat.vi"("Real Input Array"=w365) -> ("DB Output Array"=w367:u8[])  [unwired: 10 in]
        n272 = call "DB_Write.vi"("Input Params"=T18 {"Address IP"="192.168.10.80", "Rack"=0, "Slot "=0, "DB Number"=12, "Start"=56, "Amount"=32, "Word Length"=2}, "Array"=w367) -> ()  [unwired: 13 in, 1 out]
      }
      frame "PROC OK CHECK" {
        n273 = property on="PROC OK" class="Arr (strict)"() -> ("Value"=w382:bool[])  [unwired: 2 in, 2 out]
        n274 = And Array Elements(Boolean array=w382) -> (logical AND=w386:bool)
        n275 = Not(x=w386) -> (.not. x?=w385:bool)
        n276 = property on="PROC NOK" class="Bool (strict)"("Value"=w385) -> ()  [unwired: 2 in, 2 out]
        n277 = case shown="True" w385 {
          tunnel: w384 -> [w388 w391]
          tunnel: [w388 w390] -> w383
          frame False {
            n278 = property on="Running" class="Bool (strict)"() -> ("Value"=w387:bool)  [unwired: 2 in, 2 out]
            n279 = case shown="True" w387 {
              frame False {
              }
              frame True {
                n280 = property on="RUN Button" class="Bool (strict)"("DisabledEnum"=T19."Enabled" ("Disabled")) -> ()  [unwired: 2 in, 2 out]
              }
            }
          }
          frame True {
            n281 = call "Enqueue Message (Single).vi"("Error In"=w391, "Message Position"=Message_Queue_Element_Position."Front", "State Machine Message"=State_Machine_Message."PROC NOK") -> ("Error Out"=w390:errorcluster)  [unwired: 8 in]
          }
        }
      }
      frame "PROC NOK" {
        n282 = property on="RUN Button" class="Bool (strict)"("DisabledEnum"=T19."Disabled and Grayed Out" ("Disabled")) -> ()  [unwired: 2 in, 2 out]
        n283 = property on="PROC OK" class="Arr (strict)"() -> ("Value"=w394:bool[])  [unwired: 2 in, 2 out]
        n284 = To Variant(anything=w394) -> (Variant=w398:variant)
        n285 = call "UpdateProcNok.vi"("Error In"=w397, "Data"=w398) -> ("Error Out"=w396:errorcluster)  [unwired: 9 in]
        n286 = property on="Status" class="Enum (strict)"("Value"=Status."PROCNOK ACTIVE" ("Status")) -> ()  [unwired: 2 in, 2 out]
      }
      frame "ALARM CHECK" {
        n287 = property on="ALARMS" class="Arr (strict)"() -> ("Value"=w403:bool[])  [unwired: 2 in, 2 out]
        n288 = Or Array Elements(Boolean array=w403) -> (logical OR=w400:bool)
        n289 = property on="ALARM" class="Bool (strict)"("Value"=w400) -> ()  [unwired: 2 in, 2 out]
        n290 = case shown="True" w400 {
          tunnel: w402 -> [w404 w406]
          tunnel: [w404 w405] -> w401
          frame False {
          }
          frame True {
            n291 = call "Enqueue Message (Single).vi"("Error In"=w406, "Message Position"=Message_Queue_Element_Position."Front", "State Machine Message"=State_Machine_Message."ALARM ACTIVE") -> ("Error Out"=w405:errorcluster)  [unwired: 8 in]
          }
        }
      }
      frame "ALARM ACTIVE" {
        n292 = property on="ALARMS" class="Arr (strict)"() -> ("Value"=w410:bool[])  [unwired: 2 in, 2 out]
        n293 = To Variant(anything=w410) -> (Variant=w409:variant)
        n294 = property on="RUN Button" class="Bool (strict)"("DisabledEnum"=T19."Disabled and Grayed Out" ("Disabled")) -> ()  [unwired: 2 in, 2 out]
        n295 = call "UpdateAlarms.vi"("Error In"=w412, "Data"=w409) -> ("Error Out"=w411:errorcluster)  [unwired: 9 in]
        n296 = property on="Status" class="Enum (strict)"("Value"=Status."ALARMS ACTIVE" ("Status")) -> ()  [unwired: 2 in, 2 out]
      }
      frame "CHECKS" {
        # "- Send/Receive database changes to/from PLC\n- Update IO and other readings\n-"
        n297 = property on="ENTER SN" class="Str"() -> ("Value"=w463:string)  [unwired: 2 in, 2 out]
        n298 = property on="BADGE NUMBER" class="Str"() -> ("Value"=w456:string)  [unwired: 2 in, 2 out]
        n299 = property on="Running" class="Bool (strict)"() -> ("Value"=w424:bool)  [unwired: 2 in, 2 out]
        n300 = Equal?(x=w463, y="") -> (x = y?=w461:bool)
        n301 = Equal?(x=w463, y="XXXXX-XX") -> (x = y?=w460:bool)
        n302 = Equal?(x=w456, y="") -> (x = y?=w454:bool)
        n303 = property on="Sched Loaded" class="Bool (strict)"() -> ("Value"=w466:bool)  [unwired: 2 in, 2 out]
        n304 = Or(x=w461, y=w460) -> (x .or. y?=w459:bool)
        n305 = Not(x=w454) -> (.not. x?=w453:bool)
        n306 = case shown="True" w424 {
          frame False {
          }
          frame True {
            n307 = call "DB_Read.vi"("Input Params"=T21 {"Address IP"="192.168.10.80", "Rack"=0, "Slot "=0, "DB Number"=14, "Start"=4, "Amount"=2}) -> (1:w473:string, "Data"=w481:u8[])  [unwired: 8 in, 1 out]
            n308 = call "PLCtoGUIint.vi"("DB Val Qty"=u16 1, "DB Input Vals"=w481) -> ("RealValue"=w479:i16[])  [unwired: 9 in]
            n309 = Index Array(array=w479, index=0) -> (element=w475:i16)
            n310 = property on="PLC CURRENT STEP" class="DigNum (strict)"("Value"=w475) -> ()  [unwired: 2 in, 2 out]
            n311 = property on="CURRENT STEP" class="DigNum (strict)"() -> ("Value"=w476:u16)  [unwired: 2 in, 2 out]
            n312 = Not Equal?(x=w475, y=w476) -> (x != y?=w472:bool)
            n313 = Equal?(x=w473, y="No Error") -> (x = y?=w471:bool)
            n314 = And(x=w472, y=w471) -> (x .and. y?=w470:bool)
            n315 = case shown="True" w470 {
              frame False {
              }
              frame True {
                n316 = call "Enqueue Message (Single).vi"("Message Position"=Message_Queue_Element_Position."Front", "State Machine Message"=State_Machine_Message."PLC Step Change") -> ()  [unwired: 9 in, 1 out]
              }
            }
          }
        }
        n317 = Not(x=w459) -> (.not. x?=w458:bool)
        n318 = property on="Tube Loaded" class="Bool (strict)"() -> ("Value"=w469:bool)  [unwired: 2 in, 2 out]
        n319 = property on="PROC OK" class="Arr (strict)"() -> ("Value"=w468:bool[])  [unwired: 2 in, 2 out]
        n320 = property on="PROC OK" class="Arr (strict)"() -> ("Value"=w416:bool[])  [unwired: 2 in, 2 out]
        n321 = Replace Array Subset(array=w468, new element #1=w469, index #1=5 ("index"), new element #2=w466, index #2=3 ("index"), new element #3=w458, index #3=1 ("index"), new element #4=w453, index #4=7 ("index")) -> (w447:bool[])
        n322 = call "GUItoPLCBoolArray.vi"("Input Array"=w416) -> ("DB Array"=w415:u8[])  [unwired: 10 in]
        n323 = property on="PROC OK" class="Arr (strict)"("Value"=w447) -> ()  [unwired: 2 in, 2 out]
        n324 = And Array Elements(Boolean array=w447) -> (logical AND=w450:bool)
        n325 = vi-ref "QSM - Alarms.lvlib:ALARMS.vi"() -> (w446:refnum<vi>)
        n326 = Not(x=w450) -> (.not. x?=w451:bool)
        n327 = call "DB_Write.vi"("Input Params"=T18 {"Address IP"="192.168.10.80", "Rack"=0, "Slot "=1, "DB Number"=25, "Start"=0, "Amount"=4, "Word Length"=2}, "Array"=w415) -> ("Status"=→"Status 2":string)  [unwired: 13 in]
        n328 = vi-ref "QSM - IODocs.lvlib:IO Docs.vi"() -> (w445:refnum<vi>)
        n329 = case shown="True" w450 {
          frame False {
            n330 = property on="RUN Button" class="Bool (strict)"("DisabledEnum"=T19."Disabled and Grayed Out" ("Disabled")) -> ()  [unwired: 2 in, 2 out]
          }
          frame True {
            n331 = property on="Running" class="Bool (strict)"() -> ("Value"=w493:bool)  [unwired: 2 in, 2 out]
            n332 = case shown="False" w493 {
              frame False {
                n333 = property on="RUN Button" class="Bool (strict)"("DisabledEnum"=T19."Enabled" ("Disabled")) -> ()  [unwired: 2 in, 2 out]
              }
              frame True {
              }
            }
          }
        }
        n334 = property class="VI"(reference=w446) -> ("Exec.State"=w448:T27)  [unwired: 1 in, 2 out]
        n335 = property class="VI"(reference=w445) -> ("Exec.State"=w444:T27)  [unwired: 1 in, 2 out]
        n336 = property on="PROC NOK" class="Bool (strict)"("Value"=w451) -> ()  [unwired: 2 in, 2 out]
        n337 = case shown="\"Running\"" w448 {
          frame "Bad", Default {
          }
          frame "Idle" {
          }
          frame "Run top level" {
          }
          frame "Running" {
            n338 = property on="PROC OK" class="Arr (strict)"() -> ("Value"=w489:bool[])  [unwired: 2 in, 2 out]
            n339 = property on="ALARMS" class="Arr (strict)"() -> ("Value"=w488:bool[])  [unwired: 2 in, 2 out]
            n340 = To Variant(anything=w489) -> (Variant=w491:variant)
            n341 = To Variant(anything=w488) -> (Variant=w490:variant)
            n342 = call "UpdateProcNok.vi"("Data"=w491) -> ()  [unwired: 10 in, 1 out]
            n343 = call "UpdateAlarms.vi"("Data"=w490) -> ()  [unwired: 10 in, 1 out]
          }
        }
        n344 = call "DB_Read.vi"("Input Params"=T21 {"Address IP"="192.168.10.80", "Rack"=0, "Slot "=1, "DB Number"=15, "Start"=0, "Amount"=4}) -> ("Data"=w421:u8[])  [unwired: 8 in, 2 out]
        n345 = case shown="\"Running\"" w444 {
          frame "Bad", Default {
          }
          frame "Idle" {
          }
          frame "Run top level" {
          }
          frame "Running" {
            n346 = property on="Analog IO" class="Arr (strict)"() -> ("Value"=w485:dbl[])  [unwired: 2 in, 2 out]
            n347 = property on="BIAS DIFF" class="Clust (strict)"() -> ("Value"=w487:T11)  [unwired: 2 in, 2 out]
            n348 = To Variant(anything=w485) -> (Variant=w484:variant)
            n349 = To Variant(anything=w487) -> (Variant=w486:variant)
            n350 = call "APIAIOUpdateIODOCS.vi"("Data"=w484) -> ()  [unwired: 10 in, 1 out]
            n351 = call "APIBIasDiffUpdateIODOCS.vi"("Data"=w486) -> ()  [unwired: 10 in, 1 out]
          }
        }
        n352 = call "DB_Read.vi"("Input Params"=T21 {"Address IP"="192.168.10.80", "Rack"=0, "Slot "=0, "DB Number"=8, "Start"=0, "Amount"=44}) -> ("Data"=w428:u8[])  [unwired: 8 in, 2 out]
        n353 = call "PLCtoGUIBoolArray.vi"("Read Size"=4, "DB Input Vals"=w421) -> ("array"=w419:bool[])  [unwired: 9 in]
        n354 = property on="ALARMS" class="Arr (strict)"("Value"=w419) -> ()  [unwired: 2 in, 2 out]
        n355 = Or Array Elements(Boolean array=w419) -> (logical OR=w420:bool)
        n356 = call "PLCtoGUI32bit.vi"("DB Val Qty"=u16 11, "DB Input Vals"=w428) -> ("RealValue"=w426:sgl[])  [unwired: 9 in]
        n357 = property on="ALARM" class="Bool (strict)"("Value"=w420) -> ()  [unwired: 2 in, 2 out]
        n358 = property on="Analog IO" class="Arr (strict)"("Value"=w426) -> ()  [unwired: 2 in, 2 out]
        n359 = property on="Analog IO" class="Arr (strict)"() -> ("Value"=w443:dbl[])  [unwired: 2 in, 2 out]
        n360 = Array To Cluster(array=w443) -> (cluster=w442:T28)
        n361 = Unbundle By Name(w442) -> ("Value[0]"=w438:dbl, "Value[1]"=w436:dbl, "Value[2]"=w425:dbl, "Value[3]"=w435:dbl, "Value[6]"=w434:dbl, "Value[7]"=w433:dbl, "Value[8]"=w432:dbl, "Value[9]"=w431:dbl, "Value[10]"=w430:dbl)  [unwired: 1 out]
        n362 = property on="remrdgs" class="Clust (strict)"() -> ("Value"=w439:T9)  [unwired: 2 in, 2 out]
        n363 = Bundle By Name(cluster=w439, "remKVsp"=w438, "remKVrdg"=w436, "remMAsp"=w425, "remMArdg"=w435, "remIfArdg"=w434, "G1Vsp"=w433, "G2Vsp"=w432, "G1Vrdg"=w431, "G2Vrdg"=w430) -> (w437:T9)
        n364 = property on="GXVALS" class="Clust (strict)"() -> ("Value"=w441:T10)  [unwired: 2 in, 2 out]
        n365 = Bundle By Name(cluster=w441, "G1V_SP"=w433, "G2V_SP"=w432, "G1V_RDG"=w431, "G2V_RDG"=w430) -> (w440:T10)
        n366 = property on="GXVALS" class="Clust (strict)"("Value"=w440) -> ()  [unwired: 2 in, 2 out]
        n367 = property on="remrdgs" class="Clust (strict)"("Value"=w437) -> ()  [unwired: 2 in, 2 out]
      }
      frame "Handle Error" {
        n368 = Variant To Data(type=errorcluster {"status"=FALSE, "code"=0, "source"=""} ("Error In"), Variant=w499) -> (data=w496:errorcluster, error out=w498:errorcluster)  [unwired: 1 in]
        n369 = Merge Errors(w498, w497) -> (w495:errorcluster)
        n370 = call <vilib>:"Simple Error Handler.vi"("error in (no error)"=w496) -> ()  [unwired: 4 in, 5 out]
      }
      frame "Exit" {
        n371 = call "Flush Message Queue.vi"("Error In"=w506) -> ("Error Out"=w505:errorcluster)  [unwired: 9 in, 1 out]
        n372 = call "Generate User Event.vi"("User Event Priority"=usereventprio."high priority", "Error In"=w505, "Event Handler Message"=Event_Handler_Message."Exit", "User Event Reference"=w503) -> ("Error Out"=w504:errorcluster)  [unwired: 7 in]
      }
      frame "BIAS ZER" {
        n373 = property on="BIAS" class="DigNum (strict)"("Value"=0.0) -> ()  [unwired: 2 in, 2 out]
      }
      frame "DIFF ZER" {
        n374 = property on="DIFF" class="DigNum (strict)"("Value"=0.0) -> ()  [unwired: 2 in, 2 out]
      }
      frame "DIFF TOGGLE" {
        n375 = property on="DIFF" class="DigNum (strict)"() -> ("Value"=w513:dbl)  [unwired: 2 in, 2 out]
        n376 = Negate(x=w513) -> (-x=w512:dbl)
        n377 = property on="DIFF" class="DigNum (strict)"("Value"=w512) -> ()  [unwired: 2 in, 2 out]
      }
      frame "APIProcNOKUpdate" {
        n378 = property on="PROC OK" class="Arr (strict)"() -> ("Value"=w518:bool[])  [unwired: 2 in, 2 out]
        n379 = Variant To Data(error in=w521, type=w518, Variant=w519) -> (data=w516:bool[], error out=w520:errorcluster)
        n380 = Or Array Elements(Boolean array=w516) -> (logical OR=w517:bool)
        n381 = Not(x=w516) -> (.not. x?=w515:bool[])
        n382 = property on="PROC NOK" class="Bool (strict)"("Value"=w517) -> ()  [unwired: 2 in, 2 out]
        n383 = property on="PROC OK" class="Arr (strict)"("Value"=w515) -> ()  [unwired: 2 in, 2 out]
      }
      frame "APIAlarmsUpdate" {
        n384 = property on="ALARMS" class="Arr (strict)"() -> ("Value"=w527:bool[])  [unwired: 2 in, 2 out]
        n385 = Variant To Data(error in=w529, type=w527, Variant=w528) -> (data=w526:bool[], error out=w524:errorcluster)
        n386 = Or Array Elements(Boolean array=w526) -> (logical OR=w525:bool)
        n387 = property on="ALARMS" class="Arr (strict)"("Value"=w526) -> ()  [unwired: 2 in, 2 out]
        n388 = property on="ALARM" class="Bool (strict)"("Value"=w525) -> ()  [unwired: 2 in, 2 out]
        n389 = call "DB_Write.vi"("Input Params"=T18 {"Address IP"="192.168.10.80", "Rack"=0, "Slot "=1, "DB Number"=15, "Start"=4, "Amount"=1, "Word Length"=2}, "Array"=u8[] [1]) -> ()  [unwired: 13 in, 1 out]
      }
      frame "APILimitUpdate" {
        n390 = Variant To Data(error in=w544, type=string[] [], Variant=w545) -> (data=w540:string[], error out=w543:errorcluster)
        n391 = Array Size(array=w540) -> (size(s)=w539:i32)
        n392 = Decrement(x=w539) -> (x-1=w533:i32)
        n393 = Array Subset(array=w540, index=0, length=w533) -> (w537:string[])
        n394 = Index Array(array=w540, index=w533) -> (element=w538:string)
        n395 = Fract/Exp String To Number(string=w537) -> (number=w535:dbl[])  [unwired: 3 in, 1 out]
        n396 = Decimal String To Number(string=w538, default (0L)=u32 0 ("default (0 I32)")) -> (number=w534:u32)  [unwired: 1 in, 1 out]
        n397 = Build Array (concatenate)(w535, w534) -> (w530:dbl[])
        n398 = property on="LIMITS" class="Arr (strict)"("Value"=w530) -> ()  [unwired: 2 in, 2 out]
        n399 = call "GUItoPLCfloat.vi"("Real Input Array"=w530) -> ("DB Output Array"=w531:u8[])  [unwired: 10 in]
        n400 = call "DB_Write.vi"("Input Params"=T18 {"Address IP"="192.168.10.80", "Rack"=0, "Slot "=0, "DB Number"=6, "Start"=0, "Amount"=160, "Word Length"=2}, "Array"=w531) -> ()  [unwired: 13 in, 1 out]
      }
      frame "APIOperatorUpdate" {
        n401 = Variant To Data(error in=w560, type=string[] [], Variant=w561) -> (data=w554:string[], error out=w559:errorcluster)
        n402 = Index Array(array=w554, index #1=0 ("index"), index #2=1 ("index"), index #3=2 ("index")) -> (element #1=w548:string, element #2=w553:string, element #3=w552:string)
        n403 = Decimal String To Number(string=w552, default (0L)=u16 0 ("default (0 I32)")) -> (number=w549:u16)  [unwired: 1 in, 1 out]
        n404 = property on="ENTER OP" class="Str"("Value"=w548) -> ()  [unwired: 2 in, 2 out]
        n405 = property on="BADGE NUMBER" class="Str"("Value"=w548) -> ()  [unwired: 2 in, 2 out]
        n406 = Bundle By Name(cluster=T14 {"Badge Number"="", "Name"="", "Access"=enum.""} ("User Creds"), "Badge Number"=w548, "Name"=w553, "Access"=w549) -> (w550:T14)
        n407 = property on="User Creds" class="Clust (strict)"("Value"=w550) -> ()  [unwired: 2 in, 2 out]
        n408 = Greater?(x=w549, y=u16 1) -> (0:w563:bool)
        n409 = case shown="True" w563 {
          frame False {
            n410 = property on="Editor Button" class="Bool"("DisabledEnum"=T19."Disabled and Grayed Out" ("Disabled")) -> ()  [unwired: 2 in, 2 out]
            n411 = property on="Security Button" class="Bool (strict)"("DisabledEnum"=T19."Disabled and Grayed Out" ("Disabled")) -> ()  [unwired: 2 in, 2 out]
          }
          frame True {
            n412 = property on="Editor Button" class="Bool"("DisabledEnum"=T19."Enabled" ("Disabled")) -> ()  [unwired: 2 in, 2 out]
            n413 = property on="Security Button" class="Bool (strict)"("DisabledEnum"=T19."Enabled" ("Disabled")) -> ()  [unwired: 2 in, 2 out]
          }
        }
        n414 = property on="Status" class="Enum (strict)"("Value"=Status."USER SIGNED ON" ("Status")) -> ()  [unwired: 2 in, 2 out]
      }
      frame "APIAnalogIOUpdate" {
        n415 = Variant To Data(error in=w586, type=dbl[] [], Variant=w587) -> (data=w578:dbl[], error out=w582:errorcluster)
        n416 = property on="AIO Array Temp" class="Arr (strict)"(error in=w582, "Value"=w578) -> (error out=w579:errorcluster)  [unwired: 1 in, 1 out]
        n417 = property on="Analog IO" class="Arr (strict)"() -> ("Value"=w577:dbl[])  [unwired: 2 in, 2 out]
        n418 = Decimate 1D Array(w578) -> (w576:dbl[], w584:dbl[], w583:dbl[])
        n419 = Replace Array Subset(array=w577, new element=w576, index=0) -> (w575:dbl[])
        n420 = property on="OffsetGain" class="Arr (strict)"() -> ("Value"=w571:dbl[])  [unwired: 2 in, 2 out]
        n421 = Interleave 1D Arrays(w584, w583) -> (w568:dbl[])
        n422 = property on="Analog IO" class="Arr (strict)"(error in=w579, "Value"=w575) -> (error out=w581:errorcluster)  [unwired: 1 in, 1 out]
        n423 = Replace Array Subset(array=w571, new element=w568, index=0) -> (w572:dbl[])
        n424 = property on="OffsetGain" class="Arr (strict)"(error in=w581, "Value"=w572) -> (error out=w580:errorcluster)  [unwired: 1 in, 1 out]
        n425 = call "GUItoPLCfloat.vi"("Real Input Array"=w568) -> ("DB Output Array"=w570:u8[])  [unwired: 10 in]
        n426 = call "DB_Write.vi"("Input Params"=T18 {"Address IP"="192.168.10.80", "Rack"=0, "Slot "=0, "DB Number"=12, "Start"=0, "Amount"=56, "Word Length"=2}, "Array"=w570) -> ()  [unwired: 13 in, 1 out]
      }
      frame "APIOffsetGainUpdate" {
      }
      frame "APIGXValsUpdate" {
        n427 = Variant To Data(error in=w607, type=T10 {"G1V_SP"=0.0, "G2V_SP"=0.0, "G1V_RDG"=0.0, "G2V_RDG"=0.0, "g1spoffset"=0.0, "g1spgain"=0.0, "g1rdgoffset"=0.0, "g1rdggain"=0.0, "g2spoffset"=0.0, "g2spgain"=0.0, "g2rdgoffset"=0.0, "g2rdggain"=0.0} ("GXVALS"), Variant=w608) -> (data=w604:T10, error out=w605:errorcluster)
        n428 = property on="GXVALS" class="Clust (strict)"("Value"=w604) -> ()  [unwired: 2 in, 2 out]
        n429 = Cluster To Array(cluster=w604) -> (array=w599:dbl[])
        n430 = Array Subset(array=w599, index=0, length=4) -> (w592:dbl[])
        n431 = Array Subset(array=w599, index=4, length=8) -> (w590:dbl[])
        n432 = property on="Analog IO" class="Arr (strict)"() -> ("Value"=w593:dbl[])  [unwired: 2 in, 2 out]
        n433 = property on="OffsetGain" class="Arr (strict)"() -> ("Value"=w597:dbl[])  [unwired: 2 in, 2 out]
        n434 = Replace Array Subset(array=w593, new element=w592, index=7) -> (w595:dbl[])
        n435 = Replace Array Subset(array=w597, new element=w590, index=14) -> (w596:dbl[])
        n436 = property on="Analog IO" class="Arr (strict)"("Value"=w595) -> ()  [unwired: 2 in, 2 out]
        n437 = property on="OffsetGain" class="Arr (strict)"("Value"=w596) -> ()  [unwired: 2 in, 2 out]
        n438 = call "GUItoPLCfloat.vi"("Real Input Array"=w590) -> ("DB Output Array"=w591:u8[])  [unwired: 10 in]
        n439 = call "DB_Write.vi"("Input Params"=T18 {"Address IP"="192.168.10.80", "Rack"=0, "Slot "=0, "DB Number"=12, "Start"=56, "Amount"=32, "Word Length"=2}, "Array"=w591) -> ()  [unwired: 13 in, 1 out]
      }
      frame "APIBiasDiffUpdate" {
        n440 = Variant To Data(error in=w612, type=T11 {"BIAS"=0.0, "BIAS_ZER"=FALSE, "DIFF_ZER"=FALSE, "DIFF_TOGGLE"=FALSE, "DIFF"=0.0} ("BIAS DIFF"), Variant=w613) -> (data=w610:T11, error out=w611:errorcluster)
        n441 = property on="BIAS DIFF" class="Clust (strict)"("Value"=w610) -> ()  [unwired: 2 in, 2 out]
      }
      frame "API Update Selected Tube" {
        n442 = Variant To Data(error in=w626, type=u32[] [], Variant=w625) -> (data=w622:u32[], error out=w624:errorcluster)
        n443 = Index Array(array=w622, index #1=0 ("index"), index #2=1 ("index")) -> (element #1=w619:u32, element #2=w618:u32)
        n444 = Number To Boolean Array(number=w618) -> (Boolean array=w617:bool[])
        n445 = Or Array Elements(Boolean array=w617) -> (logical OR=w616:bool)
        n446 = Greater Than 0?(x=w619) -> (x > 0?=w627:bool)
        n447 = case shown="True" w627 {
          frame False {
            n448 = property on="sched sel Button" class="Bool (strict)"("DisabledEnum"=T19."Disabled and Grayed Out" ("Disabled")) -> ()  [unwired: 2 in, 2 out]
          }
          frame True {
            n449 = property on="sched sel Button" class="Bool (strict)"("DisabledEnum"=T19."Enabled" ("Disabled")) -> ()  [unwired: 2 in, 2 out]
          }
        }
        n450 = call "XML Parser Tubes.vi"("error in (no error)"=w624) -> ("error out"=w615:errorcluster, "output array"=w628:string[])  [unwired: 9 in]
        n451 = property on="Tube Loaded" class="Bool (strict)"("Value"=w616) -> ()  [unwired: 2 in, 2 out]
        n452 = case shown="True" w616 {
          tunnel: w619 -> [_ w634]
          tunnel: w628 -> [_ w631]
          frame False {
          }
          frame True {
            n453 = Decrement(x=w634) -> (x-1=w632:u32)
            n454 = property on="TUBE" class="DigNum (strict)"("Value"=w634) -> ()  [unwired: 2 in, 2 out]
            n455 = for {
              N: 9 -> [_]
              tunnel: w632 -> [w639]
              tunnel: w631 -> [w635]
              i -> [w636]
              n456 = Multiply(x=31, y=w636) -> (x*y=w640:i32)
              n457 = Add(x=w640, y=w639) -> (x+y=w641:u32)
              n458 = Index Array(array=w635, index=w641) -> (element=w638:string)
              n459 = case shown="8" w636 {
                tunnel: w638 -> [w642 w645 w646 w649 w652 w655 w660 w662 w665]
                frame 0, Default {
                  n460 = property on="NAME" class="Str"("Value"=w642) -> ()  [unwired: 2 in, 2 out]
                }
                frame 1 {
                  n461 = Decimal String To Number(string=w645, default (0L)=0.0 ("RTC")) -> (number=w644:dbl)  [unwired: 1 in, 1 out]
                  n462 = property on="RTC" class="DigNum (strict)"("Value"=w644) -> ()  [unwired: 2 in, 2 out]
                }
                frame 2 {
                  n463 = Decimal String To Number(string=w646, default (0L)=0.0 ("RTC")) -> (number=w648:dbl)  [unwired: 1 in, 1 out]
                  n464 = property on="HS" class="DigNum (strict)"("Value"=w648) -> ()  [unwired: 2 in, 2 out]
                }
                frame 3 {
                  n465 = Decimal String To Number(string=w649, default (0L)=0.0 ("RTC")) -> (number=w651:dbl)  [unwired: 1 in, 1 out]
                  n466 = property on="T100" class="DigNum (strict)"("Value"=w651) -> ()  [unwired: 2 in, 2 out]
                }
                frame 4 {
                  n467 = Decimal String To Number(string=w652, default (0L)=0.0 ("RTC")) -> (number=w654:dbl)  [unwired: 1 in, 1 out]
                  n468 = property on="T10" class="DigNum (strict)"("Value"=w654) -> ()  [unwired: 2 in, 2 out]
                }
                frame 5 {
                  n469 = Decimal String To Number(string=w655, default (0L)=0.0 ("RTC")) -> (number=w657:dbl)  [unwired: 1 in, 1 out]
                  n470 = property on="AP%" class="DigNum (strict)"("Value"=w657) -> ()  [unwired: 2 in, 2 out]
                }
                frame 6 {
                  n471 = Decimal String To Number(string=w660, default (0L)=u32 0 ("default (0 I32)")) -> (number=w658:u32)  [unwired: 1 in, 1 out]
                  n472 = property on="schd1-30" class="DigNum (strict)"("Value"=w658) -> ()  [unwired: 2 in, 2 out]
                }
                frame 7 {
                  n473 = Decimal String To Number(string=w662, default (0L)=u32 0 ("default (0 I32)")) -> (number=w661:u32)  [unwired: 1 in, 1 out]
                  n474 = property on="schd31-60" class="DigNum (strict)"("Value"=w661) -> ()  [unwired: 2 in, 2 out]
                }
                frame 8 {
                  n475 = Decimal String To Number(string=w665, default (0L)=u32 0 ("default (0 I32)")) -> (number=w664:u32)  [unwired: 1 in, 1 out]
                  n476 = property on="schd61-80" class="DigNum (strict)"("Value"=w664) -> ()  [unwired: 2 in, 2 out]
                }
              }
            }
          }
        }
        n477 = property on="Status" class="Enum (strict)"("Value"=Status."TUBE SELECTED" ("Status")) -> ()  [unwired: 2 in, 2 out]
      }
      frame "API Update Selected Schedule" {
        n478 = Variant To Data(error in=w680, type=string[] [] ("String"), Variant=w681) -> (data=w677:string[], error out=w678:errorcluster)
        n479 = Index Array(array=w677, index #1=0 ("index"), index #2=1 ("index")) -> (element #1=w674:string, element #2=w673:string)
        n480 = Decimal String To Number(string=w673, default (0L)=u32 0 ("default (0 I32)")) -> (number=w671:u32)  [unwired: 1 in, 1 out]
        n481 = Number To Boolean Array(number=w671) -> (Boolean array=w670:bool[])
        n482 = Or Array Elements(Boolean array=w670) -> (logical OR=w669:bool)
        n483 = property on="Sched Loaded" class="Bool (strict)"("Value"=w669) -> ()  [unwired: 2 in, 2 out]
        n484 = case shown="True" w669 {
          tunnel: w674 -> [_ w709]
          tunnel: [w682 w685] -> w668
          tunnel: w678 -> [w682 w692]
          frame False {
          }
          frame True {
            w683 = u16 1 ("STARTING STEP")
            n485 = property on="Schedule" class="MCListbox (strict)"() -> ("ItemNames"=w690:string[][])  [unwired: 2 in, 2 out]
            n486 = Read from Text File(file (use dialog)=path "C:/Users/Public/Documents/Grid2093/SCHEDS/SchedNames.txt" ("path")) -> (text=w695:string)  [unwired: 3 in, 3 out]
            n487 = property on="SchedNum" class="Str"("Value"=w709) -> ()  [unwired: 2 in, 2 out]
            n488 = property on="SchedNames[]" class="Arr (strict)"() -> ("Value"=w700:string[])  [unwired: 2 in, 2 out]
            n489 = String Subset(string=w709, offset (0)=5) -> (substring=w702:string)  [unwired: 1 in]
            n490 = call <vilib>:"Delimited String to 1D String Array.vi"("delimiter"=",\n", "delimited string"=w695) -> ("string array"=→"SchedNames[]":string[])  [unwired: 9 in]
            n491 = for {
              N: 32 -> [_]
              tunnel: w690 -> [w717]
              i -> [w716]
              n492 = Index Array(array=w717, index (row)=w716, index (col)=3 ("disabled index (col)")) -> (element=w713:string)
              n493 = Index Array(array=w717, index (row)=w716, index (col)=2 ("disabled index (col)")) -> (element=w715:string)
              n494 = Decimal String To Number(string=w713) -> (number=w712:i32)  [unwired: 2 in, 1 out]
              n495 = Decimal String To Number(string=w715) -> (number=w714:i32)  [unwired: 2 in, 1 out]
              n496 = Not Equal To 0?(x=w712) -> (x != 0?=w711:bool)
              n497 = Not Equal To 0?(x=w714) -> (x != 0?=w710:bool)
              n498 = Compound Arithmetic op=AND(w710, w711) -> (w719:bool)
              n499 = case shown="True" w719 {
                tunnel: w716 -> [_ w722]
                frame False {
                }
                frame True {
                  n500 = Increment(x=w722) -> (x+1=w721:i32)
                  n501 = property on="FINAL STEP" class="DigNum (strict)"("Value"=w721) -> ()  [unwired: 2 in, 2 out]
                }
              }
            }
            n502 = call "XMLEASY.vi"("error in (no error)"=w692, "Schedule Filename"=w709) -> ("error out"=w708:errorcluster, "Sched Tag Vals (1D)"=w705:string[])  [unwired: 6 in, 2 out]
            n503 = Decimal String To Number(string=w702) -> (number=w697:i32)  [unwired: 2 in, 1 out]
            n504 = Reshape Array(w705, 21 ("dimension size"), 32 ("dimension size")) -> (w704:string[][])
            n505 = Decrement(x=w697) -> (x-1=w698:i32)
            n506 = Index Array(array=w700, index=w698) -> (element=w699:string)
            n507 = Transpose 2D Array(2D array=w704) -> (transposed array=w703:string[][])
            n508 = case shown="No Error" w708 {
              selector: w708 -> [w724 w726]
              tunnel: [w723 w726] -> w689
              tunnel: w703 -> [w725 _]
              frame No Error {
                n509 = property on="Schedule" class="MCListbox (strict)"(error in=w724, "ItemNames"=w725) -> (error out=w723:errorcluster)  [unwired: 1 in, 1 out]
              }
              frame Error {
              }
            }
            n510 = property on="SchedName" class="Str"("Value"=w699) -> ()  [unwired: 2 in, 2 out]
            n511 = property on="CURRENT STEP" class="DigNum (strict)"("Value"=w683) -> ()  [unwired: 2 in, 2 out]
            n512 = property on="FIRST STEP" class="DigNum (strict)"(error in=w689, "Value"=w683) -> (error out=w685:errorcluster)  [unwired: 1 in, 1 out]
            n513 = property on="Schedule" class="MCListbox (strict)"() -> ("ItemNames"=w686:string[][])  [unwired: 2 in, 2 out]
            n514 = Index Array(array=w686, index (row)=0) -> (element=w688:string[])  [unwired: 1 in]
            n515 = call "Schedsteptodisplay.vi"("step num"=w683, "step array"=w688) -> ("STEP VARS"=w687:T12)  [unwired: 9 in]
            n516 = property on="STEP VARS" class="Clust (strict)"("Value"=w687) -> ()  [unwired: 2 in, 2 out]
          }
        }
        n517 = property on="Status" class="Enum (strict)"("Value"=Status."SCHEDULE SELECTED" ("Status")) -> ()  [unwired: 2 in, 2 out]
      }
      frame "RunResultRetestSelect" {
        n518 = property on="Run Results" class="MCListbox (strict)"() -> ("FocusRow"=w729:i32)  [unwired: 2 in, 2 out]
        n519 = Variant To Data(error in=w731, type=w729, Variant=w732) -> (data=w728:i32, error out=w730:errorcluster)
        n520 = property on="Run Results" class="MCListbox (strict)"("FocusRow"=w728) -> ()  [unwired: 2 in, 2 out]
        n521 = Increment(x=w728) -> (x+1=w727:i32)
        n522 = property on="Retest Step" class="DigNum (strict)"("Value"=w727) -> ()  [unwired: 2 in, 2 out]
      }
      frame "Retest One" {
        n523 = property on="Retest Select" class="Arr (strict)"("Value"=bool[] [TRUE]) -> ()  [unwired: 2 in, 2 out]
        n524 = property on="Retest Select" class="Arr (strict)"() -> ("Value"=w740:bool[])  [unwired: 2 in, 2 out]
        n525 = property on="Retest Step" class="DigNum (strict)"() -> ("Value"=w736:u8)  [unwired: 2 in, 2 out]
        n526 = Boolean Array To Number(Boolean array=w740) -> (number=w738:u32)
        n527 = To Unsigned Byte Integer(number=w738) -> (unsigned 8bit integer=w734:u8)
        n528 = Build Array(w736, u8 0 ("element"), w734) -> (w739:u8[])
        n529 = call "DB_Write.vi"("Input Params"=T18 {"Address IP"="192.168.10.80", "Rack"=0, "Slot "=1, "DB Number"=40, "Start"=0, "Amount"=6, "Word Length"=2}, "Array"=w739) -> ()  [unwired: 13 in, 1 out]
        n530 = property on="Status" class="Enum (strict)"("Value"=Status."RETESTING SELECTED STEP ONLY" ("Status")) -> ()  [unwired: 2 in, 2 out]
      }
      frame "Retest End" {
        n531 = property on="Retest Select" class="Arr (strict)"("Value"=bool[] [FALSE, TRUE]) -> ()  [unwired: 2 in, 2 out]
        n532 = property on="Retest Step" class="DigNum (strict)"() -> ("Value"=w743:u8)  [unwired: 2 in, 2 out]
        n533 = property on="Retest Select" class="Arr (strict)"() -> ("Value"=w745:bool[])  [unwired: 2 in, 2 out]
        n534 = Boolean Array To Number(Boolean array=w745) -> (number=w747:u32)
        n535 = To Unsigned Byte Integer(number=w747) -> (unsigned 8bit integer=w748:u8)
        n536 = Build Array(w743, w743, w748) -> (w746:u8[])
        n537 = call "DB_Write.vi"("Input Params"=T18 {"Address IP"="192.168.10.80", "Rack"=0, "Slot "=1, "DB Number"=40, "Start"=0, "Amount"=6, "Word Length"=2}, "Array"=w746) -> ()  [unwired: 13 in, 1 out]
        n538 = property on="Status" class="Enum (strict)"("Value"=Status."RETESTING SELECTED STEP TO END" ("Status")) -> ()  [unwired: 2 in, 2 out]
      }
      frame "Print Datasheet" {
        n539 = vi-ref "DatasheetPrinter.vi"() -> (w757:refnum<vi>)
        n540 = property class="VI"(reference=w757, error in=w754) -> (error out=w762:errorcluster, "Name"=w763:string)  [unwired: 1 out]
        n541 = Open VI Reference(type specifier VI Refnum (for type only)=refnum<vi> refnum, vi path=w763, options=128, error in (no error)=w762) -> (vi reference=w755:refnum<vi>, error out=w761:errorcluster)  [unwired: 2 in]
        n542 = call-by-ref "Start Asynchronous Call"(reference=w755, error in=w761) -> (reference out=w759:refnum<vi>, error out=w758:errorcluster)  [unwired: 12 in]
        n543 = Close Reference(reference=w759, error in (no error)=w758) -> (error out=w753:errorcluster)
        n544 = property on="Status" class="Enum (strict)"("Value"=Status."PRINTING DATASHEET" ("Status")) -> ()  [unwired: 2 in, 2 out]
      }
      frame "FlatPanelCamera" {
      }
    }
    n545 = call "Enqueue Handle Error Message on Error.vi"("Error In"=w38) -> ("Error Out"=w37:errorcluster)  [unwired: 10 in]
  }
  n546 = while {
    shift-right: [w769] -> w24
    shift-left: w8 -> [w771]
    tunnel: [w766] -> w11
    tunnel: w10 -> [w765]
    stop <- w772 stop-if-true
    # "Event Handler"
    n547 = event shown="[25] Timeout" {
      selector: w765 -> [_ _ _ _ _ _ _ _ _ _ _ _ _ _ _ _ _ _ _ _ _ _ _ _ _ _ _ _]
      dyn-events: [_ _ _ _ _ _ _ _ _ _ _ _ _ _ _ _ _ _ _ _ _ _ _ _ _ _ _ _] -> w766
      timeout: 500 -> [_ _ _ _ _ _ _ _ _ _ _ _ _ _ _ _ _ _ _ _ _ _ _ _ _ _ _ _]
      tunnel: [_ _ _ _ _ _ _ _ _ _ _ _ _ _ _ _ _ _ _ _ _ _ _ _ _ _ w887 _] -> w772
      tunnel: w771 -> [w774 w778 w784 w787 w794 w798 w802 w806 w810 w814 w818 w822 w826 w830 w834 w838 w842 w846 w850 w855 w862 w865 w870 w874 w880 w884 _ w891]
      tunnel: [w773 w777 w783 w786 w793 w797 w801 w805 w809 w813 w817 w821 w825 w829 w833 w837 w841 w845 w849 w854 w861 w866 w869 w873 w879 w883 _ w890] -> w770
      event "Log In Button": Value Change {
        n548 = event-data() -> ()  [unwired: 1 in, 6 out]
        n549 = call "Enqueue Message (Single).vi"("Error In"=w774, "Message Position"=Message_Queue_Element_Position."Front", "State Machine Message"=State_Machine_Message."Operator Signon") -> ("Error Out"=w773:errorcluster)  [unwired: 8 in]
      }
      event "Editor Button": Value Change {
        n550 = event-data() -> ()  [unwired: 1 in, 6 out]
        n551 = call "Enqueue Message (Single).vi"("Error In"=w778, "Message Position"=Message_Queue_Element_Position."Front", "State Machine Message"=State_Machine_Message."Editor") -> ("Error Out"=w777:errorcluster)  [unwired: 8 in]
      }
      event "Security Button": Value Change {
        n552 = event-data() -> ()  [unwired: 1 in, 6 out]
        n553 = call "Enqueue Message (Single).vi"("Error In"=w784, "Message Position"=Message_Queue_Element_Position."Front", "State Machine Message"=State_Machine_Message."Security") -> ("Error Out"=w783:errorcluster)  [unwired: 8 in]
      }
      event "Load Tube Button": Value Change {
        n554 = event-data() -> ("NewVal"=w785:bool)  [unwired: 1 in, 5 out]
        n555 = case shown="True" w785 {
          tunnel: w787 -> [w788 w790]
          tunnel: [w788 w789] -> w786
          frame False {
          }
          frame True {
            n556 = call "Enqueue Message (Single).vi"("Error In"=w790, "Message Position"=Message_Queue_Element_Position."Front", "State Machine Message"=State_Machine_Message."Select Tube") -> ("Error Out"=w789:errorcluster)  [unwired: 8 in]
          }
        }
      }
      event "sched sel Button": Value Change {
        n557 = event-data() -> ()  [unwired: 1 in, 6 out]
        n558 = call "Enqueue Message (Single).vi"("Error In"=w794, "Message Position"=Message_Queue_Element_Position."Front", "State Machine Message"=State_Machine_Message."Select Sched") -> ("Error Out"=w793:errorcluster)  [unwired: 8 in]
      }
      event "View Sched Button": Value Change {
        n559 = event-data() -> ()  [unwired: 1 in, 6 out]
        n560 = call "Enqueue Message (Single).vi"("Error In"=w798, "Message Position"=Message_Queue_Element_Position."Front", "State Machine Message"=State_Machine_Message."View Sched") -> ("Error Out"=w797:errorcluster)  [unwired: 8 in]
      }
      event "IO/DOCS Button": Value Change {
        n561 = event-data() -> ()  [unwired: 1 in, 6 out]
        n562 = call "Enqueue Message (Single).vi"("Error In"=w802, "Message Position"=Message_Queue_Element_Position."Front", "State Machine Message"=State_Machine_Message."View IO/DOCS") -> ("Error Out"=w801:errorcluster)  [unwired: 8 in]
      }
      event Value Change {
        n563 = event-data() -> ()  [unwired: 1 in, 6 out]
        n564 = call "Enqueue Message (Single).vi"("Error In"=w806, "Message Position"=Message_Queue_Element_Position."Front", "State Machine Message"=State_Machine_Message."New Gx Val") -> ("Error Out"=w805:errorcluster)  [unwired: 8 in]
      }
      event "LIMITS Button": Value Change {
        n565 = event-data() -> ()  [unwired: 1 in, 6 out]
        n566 = call "Enqueue Message (Single).vi"("Error In"=w810, "Message Position"=Message_Queue_Element_Position."Front", "State Machine Message"=State_Machine_Message."View LIMITS") -> ("Error Out"=w809:errorcluster)  [unwired: 8 in]
      }
      event "ALARMS BUtton": Value Change {
        n567 = event-data() -> ()  [unwired: 1 in, 6 out]
        n568 = call "Enqueue Message (Single).vi"("Error In"=w814, "Message Position"=Message_Queue_Element_Position."Front", "State Machine Message"=State_Machine_Message."View ALARMS") -> ("Error Out"=w813:errorcluster)  [unwired: 8 in]
      }
      event "FIRST STEP": Value Change {
        n569 = event-data() -> ()  [unwired: 1 in, 6 out]
        n570 = call "Enqueue Message (Single).vi"("Error In"=w818, "Message Position"=Message_Queue_Element_Position."Front", "State Machine Message"=State_Machine_Message."Start Step Change") -> ("Error Out"=w817:errorcluster)  [unwired: 8 in]
      }
      event "PLC CURRENT STEP": Value Change {
        n571 = event-data() -> ()  [unwired: 1 in, 6 out]
        n572 = call "Enqueue Message (Single).vi"("Error In"=w822, "Message Position"=Message_Queue_Element_Position."Front", "State Machine Message"=State_Machine_Message."PLC Step Change") -> ("Error Out"=w821:errorcluster)  [unwired: 8 in]
      }
      event "ENTER SN": Value Change {
        n573 = event-data() -> ()  [unwired: 1 in, 6 out]
        n574 = call "Enqueue Message (Single).vi"("Error In"=w826, "Message Position"=Message_Queue_Element_Position."Front", "State Machine Message"=State_Machine_Message."New Serial Number") -> ("Error Out"=w825:errorcluster)  [unwired: 8 in]
      }
      event "RUN Button": Value Change {
        n575 = event-data() -> ()  [unwired: 1 in, 6 out]
        n576 = call "Enqueue Message (Single).vi"("Error In"=w830, "Message Position"=Message_Queue_Element_Position."Front", "State Machine Message"=State_Machine_Message."RUN Initiated") -> ("Error Out"=w829:errorcluster)  [unwired: 8 in]
      }
      event "RESET Button": Value Change {
        n577 = event-data() -> ()  [unwired: 1 in, 6 out]
        n578 = call "Enqueue Message (Single).vi"("Error In"=w834, "Message Position"=Message_Queue_Element_Position."Front", "State Machine Message"=State_Machine_Message."RESET Initiated") -> ("Error Out"=w833:errorcluster)  [unwired: 8 in]
      }
      event "PROC OK": Value Change {
        n579 = event-data() -> ()  [unwired: 1 in, 6 out]
        n580 = call "Enqueue Message (Single).vi"("Error In"=w838, "Message Position"=Message_Queue_Element_Position."Front", "State Machine Message"=State_Machine_Message."PROC OK CHECK") -> ("Error Out"=w837:errorcluster)  [unwired: 8 in]
      }
      event "ALARMS": Value Change {
        n581 = event-data() -> ()  [unwired: 1 in, 6 out]
        n582 = call "Enqueue Message (Single).vi"("Error In"=w842, "Message Position"=Message_Queue_Element_Position."Front", "State Machine Message"=State_Machine_Message."ALARM CHECK") -> ("Error Out"=w841:errorcluster)  [unwired: 8 in]
      }
      event Value Change {
        n583 = event-data() -> ()  [unwired: 1 in, 6 out]
        n584 = call "Enqueue Message (Single).vi"("Error In"=w846, "Message Position"=Message_Queue_Element_Position."Front", "State Machine Message"=State_Machine_Message."BIAS ZER") -> ("Error Out"=w845:errorcluster)  [unwired: 8 in]
      }
      event Value Change {
        n585 = event-data() -> ()  [unwired: 1 in, 6 out]
        n586 = call "Enqueue Message (Single).vi"("Error In"=w850, "Message Position"=Message_Queue_Element_Position."Front", "State Machine Message"=State_Machine_Message."DIFF ZER") -> ("Error Out"=w849:errorcluster)  [unwired: 8 in]
      }
      event Value Change {
        n587 = event-data() -> ("NewVal"=w853:bool)  [unwired: 1 in, 5 out]
        n588 = case shown="True" w853 {
          tunnel: w855 -> [w856 w858]
          tunnel: [w856 w857] -> w854
          frame False {
          }
          frame True {
            n589 = call "Enqueue Message (Single).vi"("Error In"=w858, "Message Position"=Message_Queue_Element_Position."Front", "State Machine Message"=State_Machine_Message."DIFF TOGGLE") -> ("Error Out"=w857:errorcluster)  [unwired: 8 in]
          }
        }
      }
      event "RetestOne": Value Change {
        n590 = event-data() -> ()  [unwired: 1 in, 6 out]
        n591 = call "Enqueue Message (Single).vi"("Error In"=w862, "Message Position"=Message_Queue_Element_Position."Front", "State Machine Message"=State_Machine_Message."Retest One") -> ("Error Out"=w861:errorcluster)  [unwired: 8 in]
      }
      event "RetestEnd": Value Change {
        n592 = event-data() -> ()  [unwired: 1 in, 6 out]
        n593 = call "Enqueue Message (Single).vi"("Error In"=w865, "Message Position"=Message_Queue_Element_Position."Front", "State Machine Message"=State_Machine_Message."Retest End") -> ("Error Out"=w866:errorcluster)  [unwired: 8 in]
      }
      event "PrintDatasheet": Value Change {
        n594 = event-data() -> ()  [unwired: 1 in, 6 out]
        n595 = call "Enqueue Message (Single).vi"("Error In"=w870, "Message Position"=Message_Queue_Element_Position."Front", "State Machine Message"=State_Machine_Message."Print Datasheet") -> ("Error Out"=w869:errorcluster)  [unwired: 8 in]
      }
      event "FPCamera_PB": Value Change {
        n596 = event-data() -> ()  [unwired: 1 in, 6 out]
        n597 = call "Enqueue Message (Single).vi"("Error In"=w874, "Message Position"=Message_Queue_Element_Position."Front", "State Machine Message"=State_Machine_Message."FlatPanelCamera") -> ("Error Out"=w873:errorcluster)  [unwired: 8 in]
      }
      event "Run Results": Double Click {
        n598 = event-data() -> ("Row"=w877:i32)  [unwired: 1 in, 8 out]
        n599 = To Variant(anything=w877) -> (Variant=w878:variant)
        n600 = call "Enqueue Message (Single).vi"("Error In"=w880, "Message Position"=Message_Queue_Element_Position."Front", "Data"=w878, "State Machine Message"=State_Machine_Message."RunResultRetestSelect") -> ("Error Out"=w879:errorcluster)  [unwired: 7 in]
      }
      event Timeout {
        # "Random number generator for \ntesting of asynchronous VI calls."
        n601 = event-data() -> ()  [unwired: 1 in, 3 out]
        n602 = call "Enqueue Message (Single).vi"("Error In"=w884, "Message Position"=Message_Queue_Element_Position."Back", "State Machine Message"=State_Machine_Message."CHECKS") -> ("Error Out"=w883:errorcluster)  [unwired: 8 in]
      }
      event User Event {
        n603 = event-data() -> ("Event Handler Message"=w888:T23)  [unwired: 1 in]
        n604 = case shown="\"Exit\"" w888 {
          tunnel: [TRUE] -> w887
          frame "Exit" {
            # "Stop Event Handler."
            # "Exit message received."
          }
        }
      }
      event "stop": Value Change {
        n605 = event-data() -> ()  [unwired: 1 in, 6 out]
        n606 = call "Enqueue Message (Single).vi"("Error In"=w891, "Message Position"=Message_Queue_Element_Position."Front", "State Machine Message"=State_Machine_Message."Exit") -> ("Error Out"=w890:errorcluster)  [unwired: 8 in]
      }
    }
    n607 = Get Date/Time In Seconds() -> (seconds since 1Jan1904=→"current time":timestamp)
    n608 = call "Enqueue Handle Error Message on Error.vi"("Error In"=w770) -> ("Error Out"=w769:errorcluster)  [unwired: 10 in]
  }
  n609 = Merge Errors(w24, w23) -> (w22:errorcluster)
  n610 = call "Destroy Message Queue.vi"("Error In"=w22) -> ("Error Out"=w14:errorcluster)  [unwired: 10 in]
  n611 = call "Unregister From User Event.vi"("Error In"=w14, "User Event Registration Reference"=w11) -> ("Error Out"=w13:errorcluster)  [unwired: 9 in]
  n612 = call "Destroy User Event.vi"("Error In"=w13, "User Event Reference"=w9) -> ("Error Out"=→"Error Out":errorcluster)  [unwired: 9 in]
  "BADGE NUMBER" <- w27
  "Op Name" <- w27
  "Access" <- u16 0 ("Access")
  "TUBE" <- w20
  "RTC" <- w20
  "HS" <- w20
  "T100" <- w20
  "T10" <- w20
  "AP%" <- w20
  "NAME" <- "XXXXXXXXXX" ("NAME")
  "schd1-30" <- w19
  "schd31-60" <- w19
  "schd61-80" <- w19
  "SchedNum" <- w18
  "SchedName" <- w18
